vi "main.vi"() -> ()   [LabVIEW 2019]
uses:
  startup_FSM.ctl
  dc_ps_FSM.ctl
  datalog.ctl
  current_ramp_FSM.ctl
  <vilib>/Analysis/6fits.llb/Curve Fitting Criteria.ctl
  <vilib>/Analysis/NI_AALPro.lvlib
  <vilib>/gmath/NI_Gmath.lvlib
panel:
  out "X":dbl[](array[numeric])=[250.0, 300.0, 350.0, 400.0, 450.0, 500.0, 550.0, 600.0, 650.0, 700.0]
  out "points":cluster{"Array":dbl[], "Mean":dbl[]}
  out "Mean":dbl[](array[numeric])
  out "NewVal 5":bool
  in  "appended path":path
  in  "?":T1(tab)
  out "Numeric":dbl min=0.0 max=1.0 step=0.005
  out "Digital Flow Measurements":waveform(dbl)(graph)
  in  "ADJUST":bool
  out "DATA LOG LED":bool
  out "DATA LOG":string
  in  "VOLTAGE":bool
  in  "RESET & CLEAR":bool
  in  "READ ERROR":bool
  in  "Next":bool
  in  "CURRENT LIMIT [A]":dbl(slide)=0.5 min=0.0 max=1.0 step=0.05 scale=0.0..1.0
  in  "OUTPUT CHANNEL":enum32{"Channel 1", "Channel 2", "Channel 3"}(radio)
  in  "STEP":dbl=0.10000000000000002 min=0.05 max=0.5 step=0.05
  out "Slide":dbl(slide) scale=0.0..100.0
  in  "CURRENT RAMP":bool
  in  "POWER SUPPLY STATUS":bool
  in  "Read Button":bool
  in  "Knob":dbl(knob) min=0.0 max=1.0 step=0.005 scale=0.0..1.0
  in  "GPIB ADDRESS":string(combo)="2"
  in  "SERIAL PORT":string(combo)="COM5"
  in  "Command Box":string(combo)
  out "SAMPLE  COUNT":dbl
  out "flow meas":dbl caption="FLOW RATE [SLPM]"
  in  "SAMP. FREQ. [HZ]":dbl=1.0 min=1.0 max=2.5 step=0.5
  in  "New Script":bool
  in  "Clear Buffer":bool
  in  "Connect Button":bool
  in  "Save As Button":bool
  in  "BAUD":string(combo)="9600" caption="BAUD RATE (BIT/S)"
  in  "Start DAQ 2":bool
  in  "Start DAQ":bool
  in  "Stop DAQ":bool
  in  "Configuration":T2={"Sampling"={"Samples per channel"=0, "Sample rate"=0.0}, "Acquisition"={"physical channels"="", "sample mode"=enum."Hardware Timed Single Point", "Min Val."=0.0, "Max Val."=0.0}}
  out "Analogue Flow Measurements":waveform(dbl)(graph)
  out "Coefficients":dbl[](array[numeric])=[-3.1117144499904428, 0.02542890920743523, -2.6853289603939732e-05, 1.2947146249008665e-08]
  in  "Show Curve":bool=TRUE
  in  "Show Points":bool=TRUE
  in  "Load Data":bool
  out "appended array":cluster{"X Values":dbl[], "Y Values":dbl[]}[](graph)=[{"X Values"=[250.0, 300.0, 350.0, 400.0, 450.0, 500.0, 550.0, 600.0, 650.0, 700.0], "Y Values"=[1.805424999999999, 2.3810990099009968, 3.0371608910891195, 3.656717821782189, 4.100871287128724, 4.4772945544554315, 4.869299504950476, 5.299580000000001, 5.624591584158401, 5.9728574999999875]}, {"X Values"=[250.00018963565154, 295.000164139512, 340.0000282955542, 385.00004256878935, 430.00026277216773, 475.00029313870596, 520.0001594137282, 565.0001288827434, 610.0004242971758, 655.0001368461951, 700.0004476537845], "Y Values"=[1.7622871059542533, 2.3768000375757894, 2.9289624170767077, 3.425856115012801, 3.874559922213396, 4.282148677197654, 4.6557018474018514, 5.0023004682122965, 5.3290247161472895, 5.642946889493036, 5.951154061007404]}]
  out "Formula":string="y =  -3.1117 + 0.0254*x - 2.6853E-5*x^2 + 1.2947E-8*x^3"
  out "MSE":dbl=0.0014069661559321211
  in  "Poly Order":i32=3 min=2 max=4 step=1
  in  "Array":bool[](array[boolean])=[FALSE, FALSE, TRUE, FALSE]
  in  "FIT Button":bool caption="Fit"
  in  "base path":path=path "C:/Users/anton/myUnisannio/magistrale/MAPI/esame/acquisizioni"
  # "OUTPUT CURRENT [A]"
  # "POWER SUPPLY \nCONTROLS"
  # "0V"
  # "12V"
  # "A"
  # "linear"
  # "exp"
  # "poly"
  # "power"
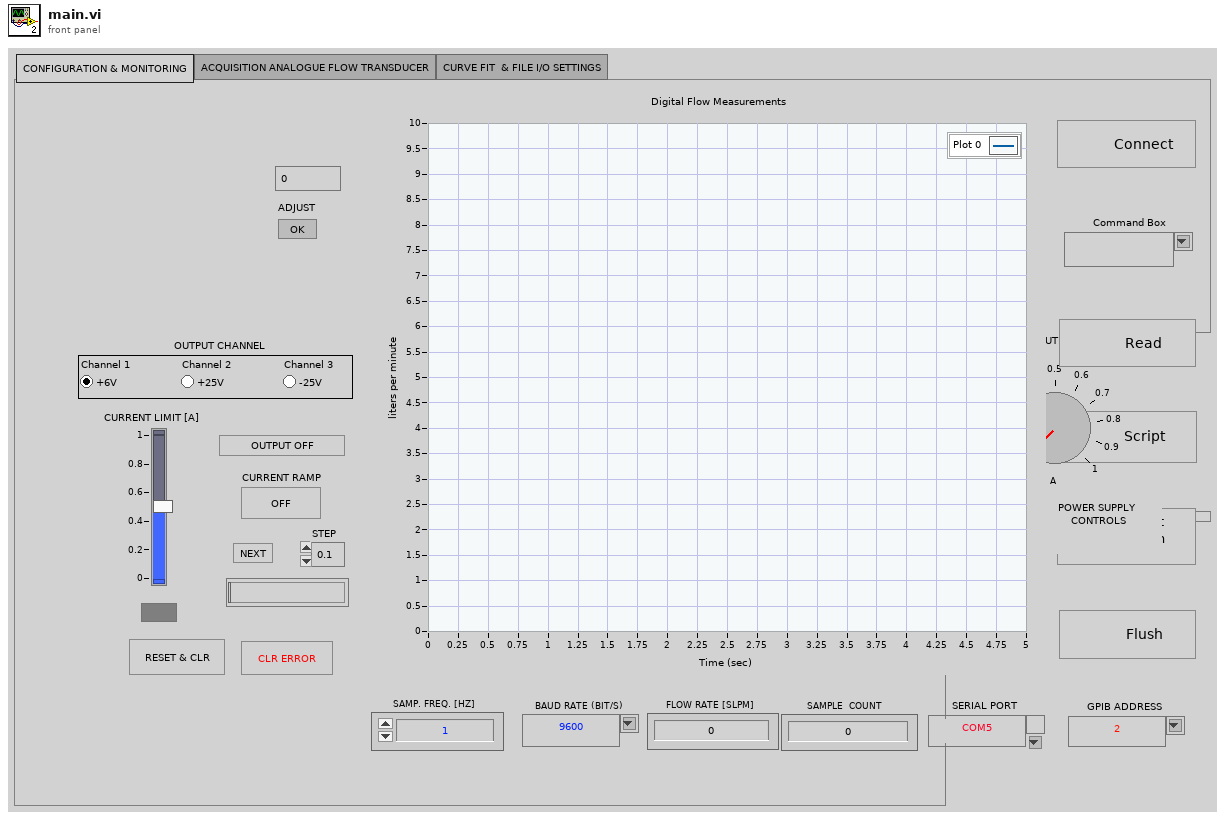
[diagram p1: front panel]
types:
  T1 = enum32{"CONFIGURATION & MONITORING", "ACQUISITION ANALOGUE FLOW TRANSDUCER", "CURVE FIT  & FILE I/O SETTINGS"}
  T2 = cluster{"Sampling":cluster{"Samples per channel":i32, "Sample rate":dbl}, "Acquisition":cluster{"physical channels":tag, "sample mode":enum16{"Finite Samples", "Continuous Samples", "Hardware Timed Single Point"}, "Min Val.":dbl, "Max Val.":dbl}}
  T3 = enum16{"", "Initialize", "Wait", "Shutdown", "Configure", "Read"}
  T4 = enum8{"Enabled", "Disabled", "Disabled and Grayed Out"}
  T5 = typedef "current_ramp_FSM.ctl" = enum16{"STATUS UPDATE", "INIT", "ERROR", "RAMP SETUP", "RAMP ENABLE", "RAMP DISABLE", "RAMP UP", "RAMP DOWN"}
  T6 = typedef "datalog.ctl" = enum16{"Error", "Read Script", "Play Script", "Changed Baud", "Changed Samp. Freq.", "Read All", "Changed Meas Unit", "Print Waveform", "Ramp Disabled", "Ramp Enabled", "Changed Ramp Step", "Changed Output Channel", "Read Error Power Supply", "Reset Power Supply", "DC Output OFF", "DC Output ON", "Connected Arduino", "Disconnected Arduino", "Disable", "Enable", "Changed Port", "Clear DL", "Changed DC Volt", "Changed Out Curr", "Stop Timer", "Start Timer", "Changed Max. Curr."}
  T7 = typedef "dc_ps_FSM.ctl" = enum16{"RESET", "VOLTAGE 12", "VOLTAGE 0", "INIT", "IDLE", "OUTPUT OFF", "OUTPUT ON", "OUT CURR", "SELECT CH", "LIMITS", "ENABLE RAMP", "RAMP UP", "RAMP DOWN", "RAMP STEP", "MEAS", "MEAS?", "ERROR", "READ ERROR", "DISABLE RAMP"}
  T8 = typedef "startup_FSM.ctl" = enum16{"IDLE", "INIT", "START MEAS", "READ", "STOP MEAS", "CHANGE BAUD", "CHANGE SAMP. FREQ.", "CHANGE PORT", "WRITE", "DISCONNECT", "CONNECT", "OUTPUT OFF", "MEAS_UNIT_L", "MEAS_UNIT_mL", "ERROR", "CLEAR BUFF", "OUTPUT ON"}
  T9 = enum16{"Linear", "Polynomial", "Exponential", "Power"}
  T10 = typedef "NI_AALPro.lvlib/Curve Fitting Criteria.ctl" = u16
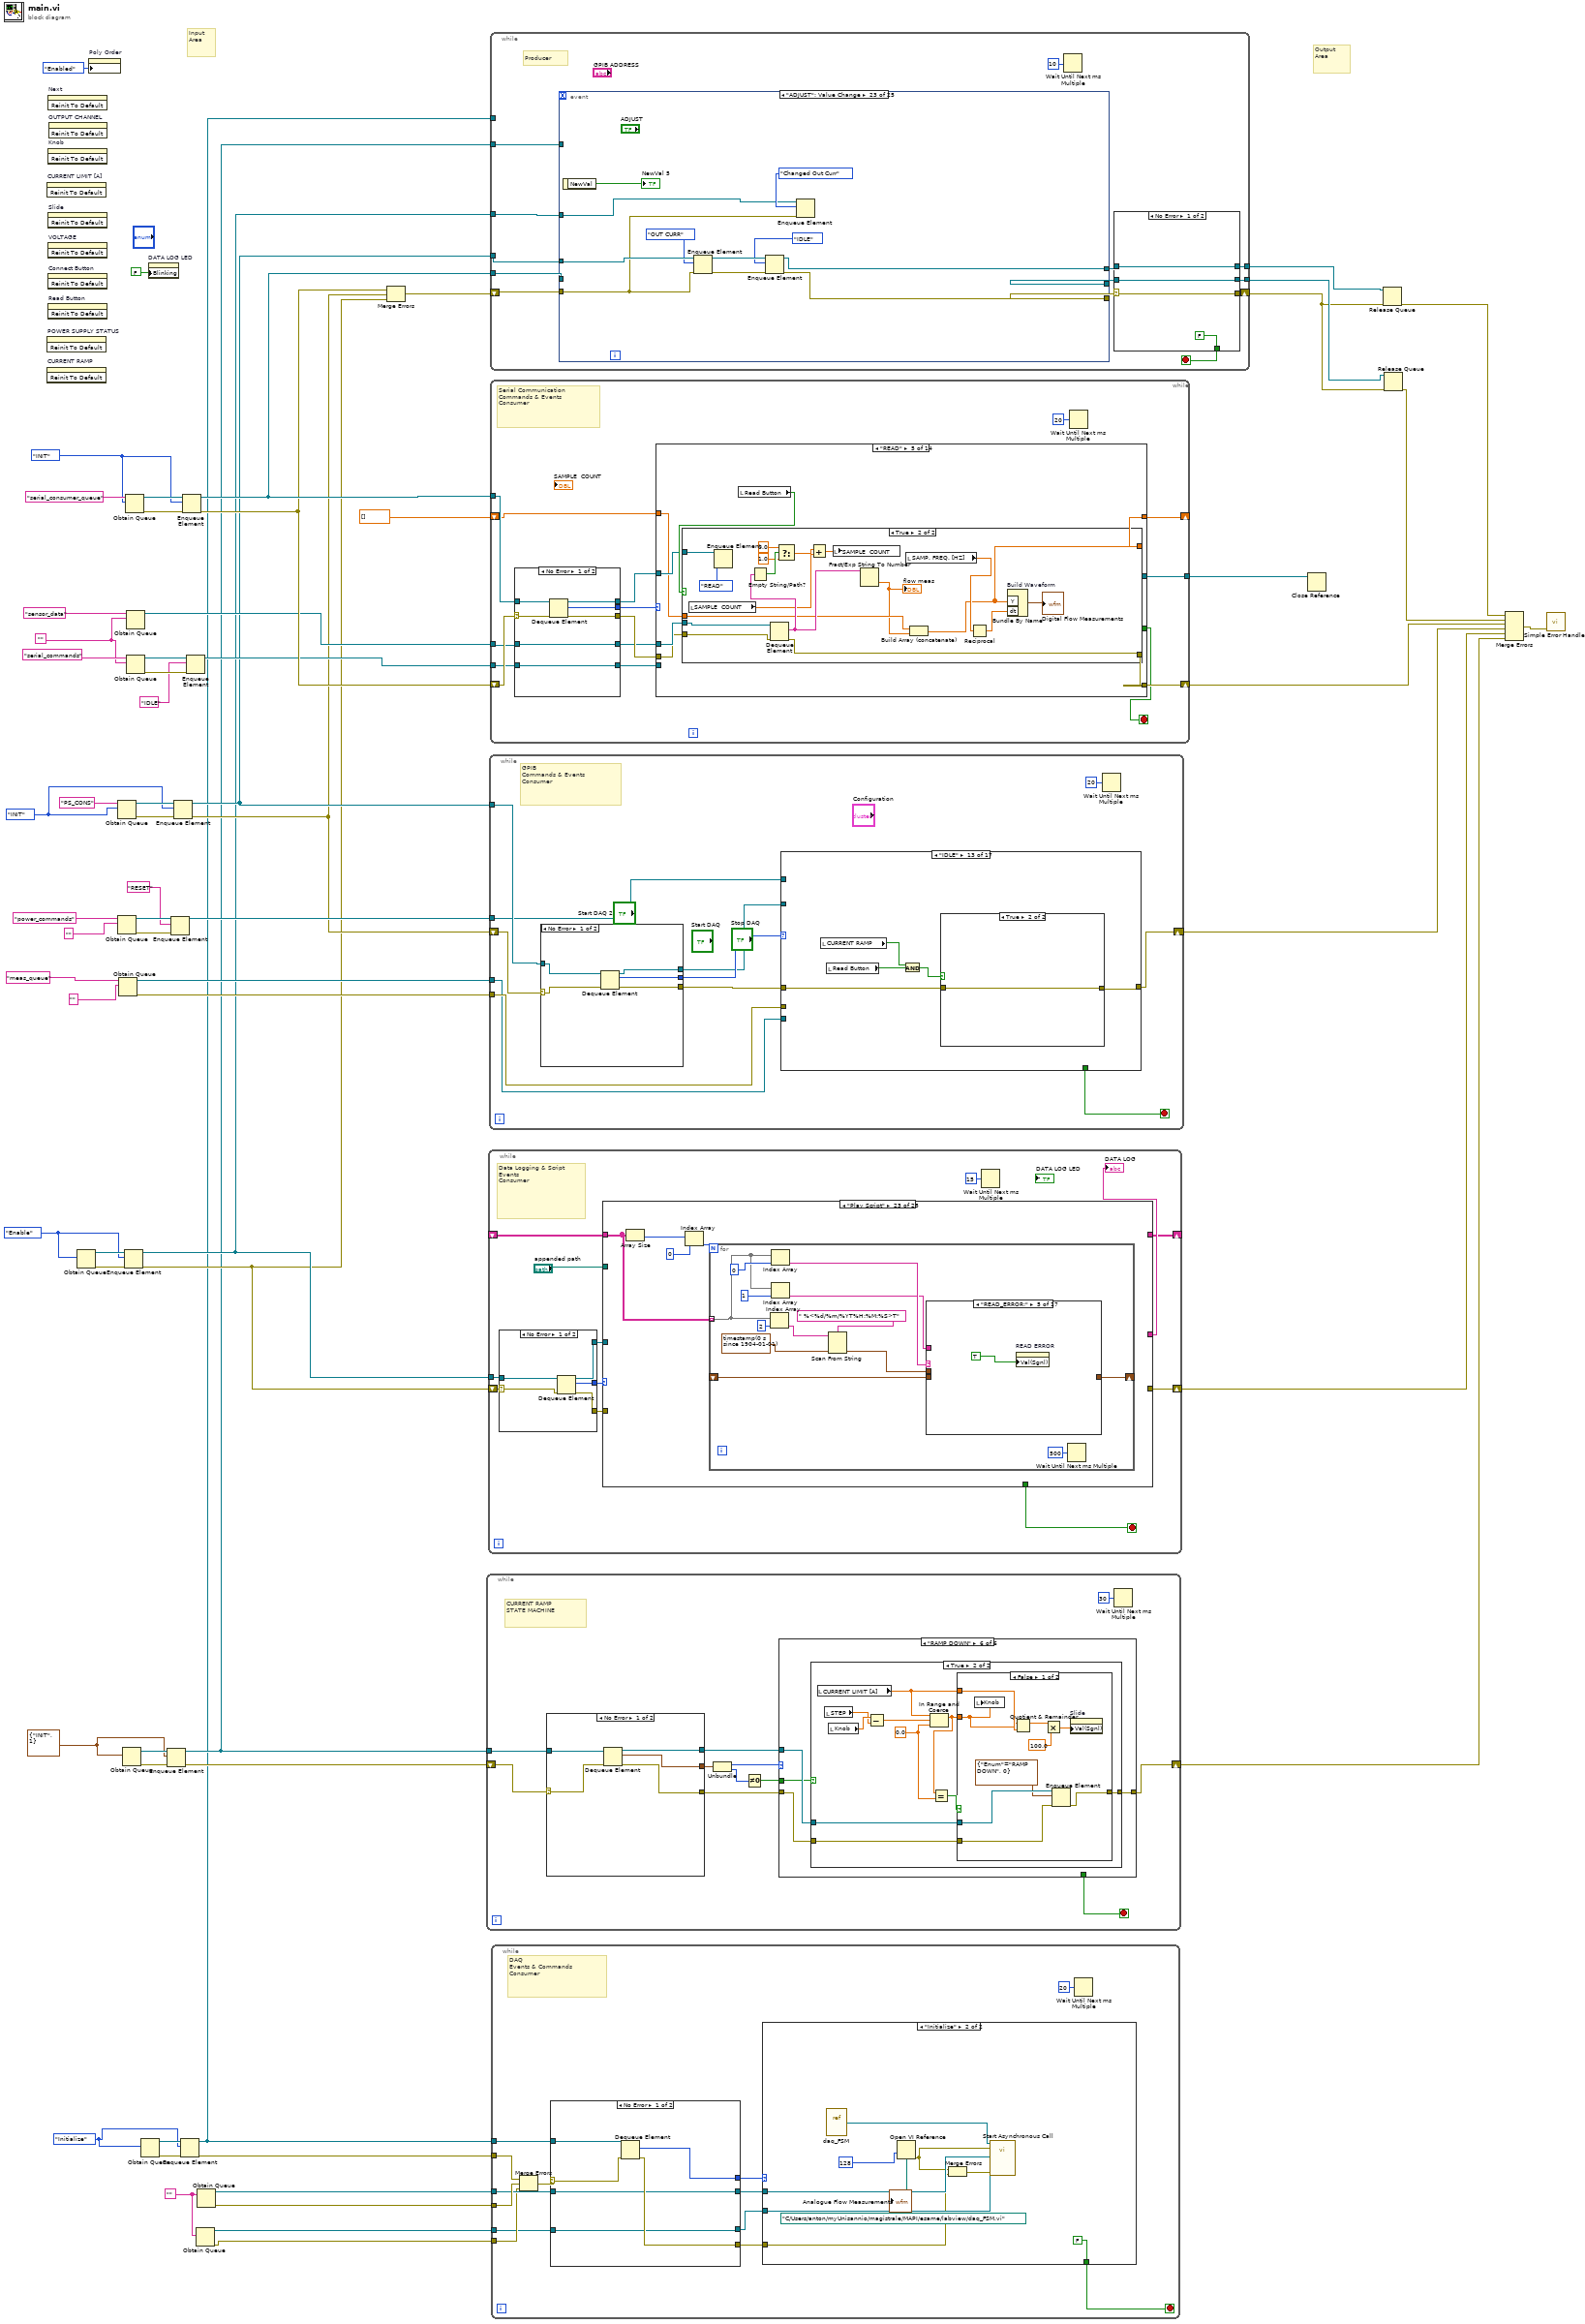
[diagram p0: block diagram]
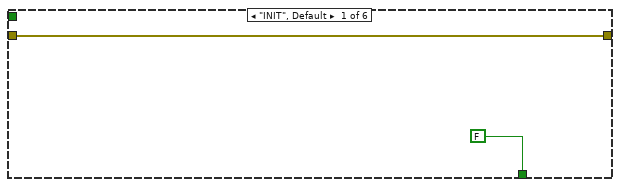
[diagram p4: hidden frame]
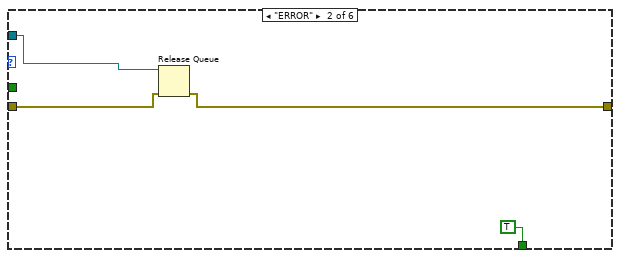
[diagram p5: hidden frame]
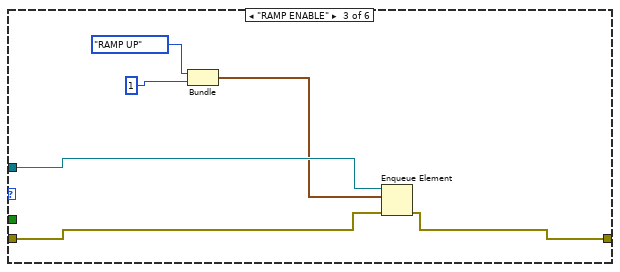
[diagram p6: hidden frame]
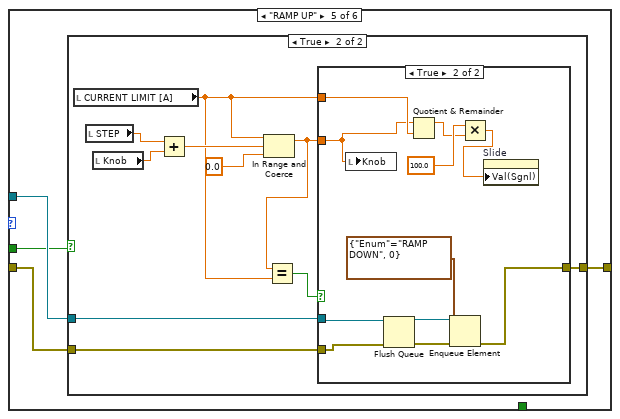
[diagram p8: hidden frame]
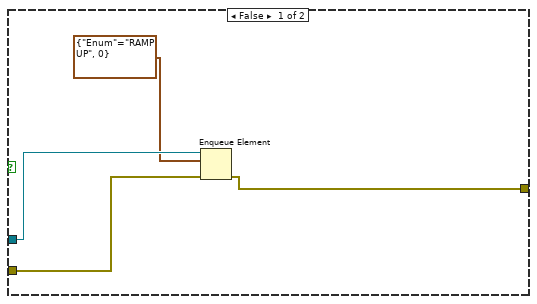
[diagram p9: hidden frame]
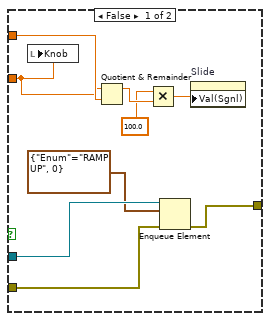
[diagram p10: hidden frame]
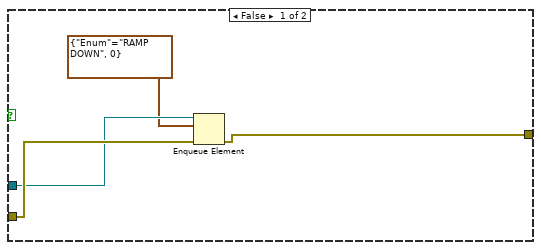
[diagram p11: hidden frame]
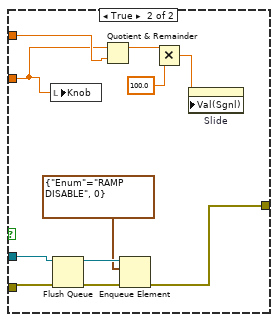
[diagram p12: hidden frame]
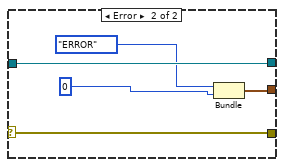
[diagram p13: hidden frame]
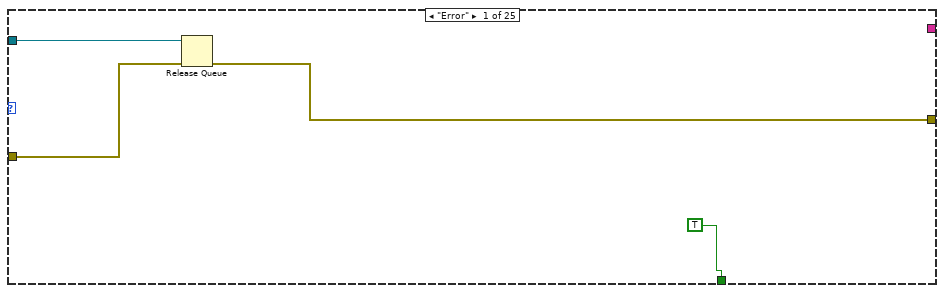
[diagram p14: hidden frame]
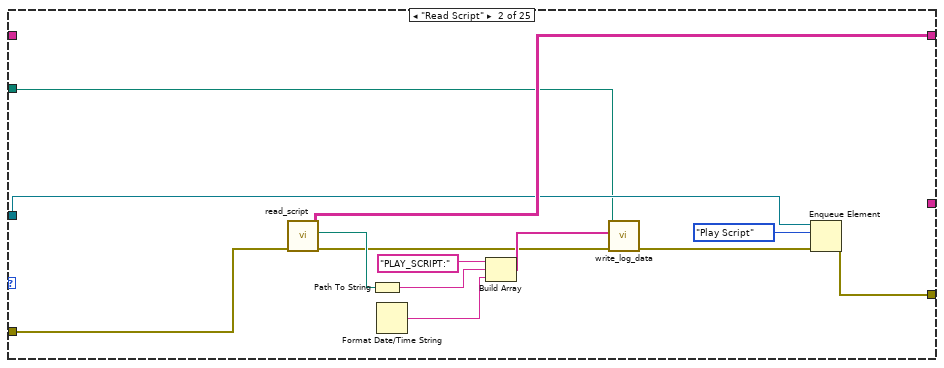
[diagram p15: hidden frame]
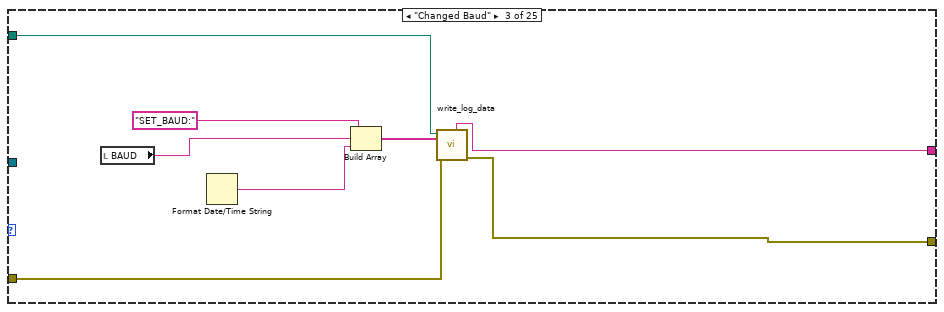
[diagram p16: hidden frame]
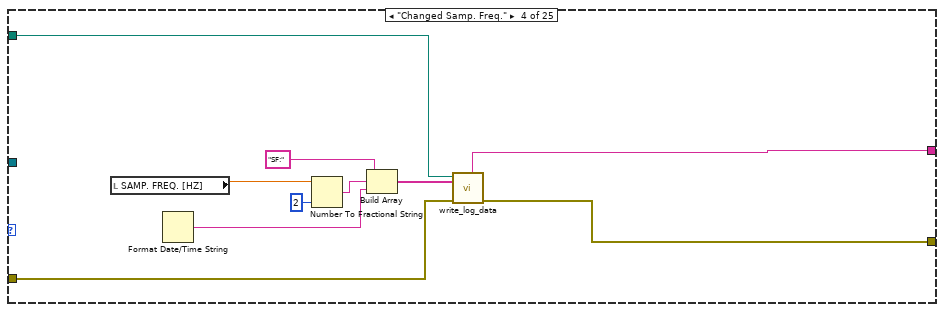
[diagram p17: hidden frame]
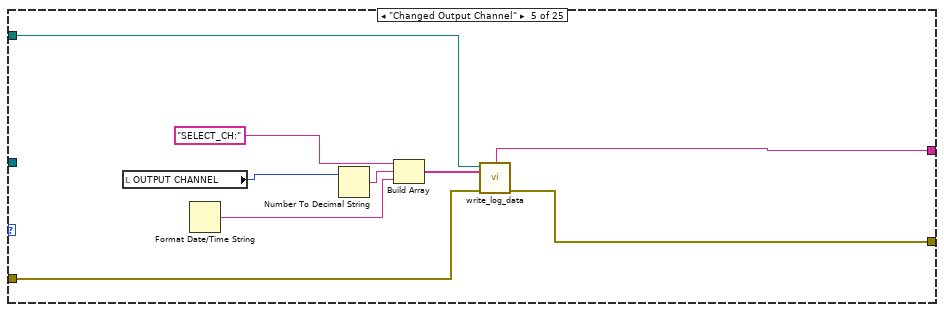
[diagram p18: hidden frame]
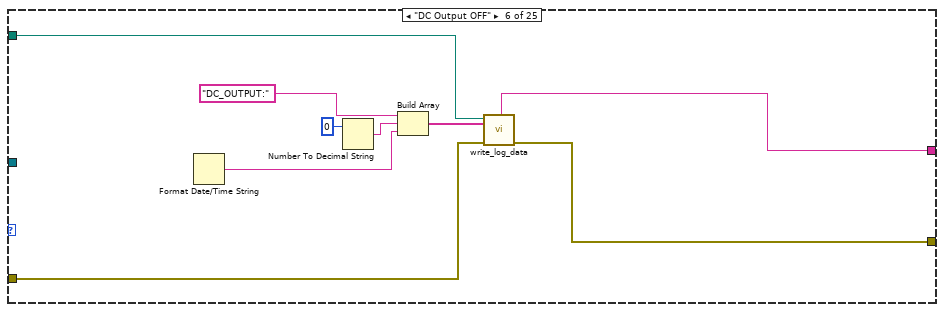
[diagram p19: hidden frame]
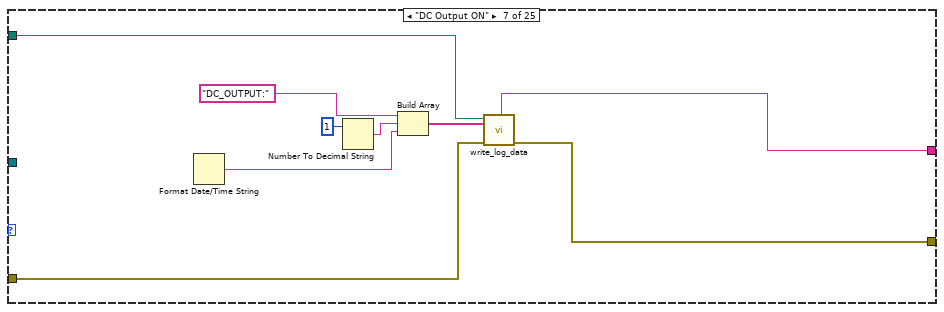
[diagram p20: hidden frame]
diagram:
  w1 = ""
  w8 = T3."Initialize" ("Enum")
  w16 = cluster{"Enum":T5, i32} {"Enum"=enum."INIT", 1} ("error constant")
  w25 = datalog."Enable" ("Enum")
  w44 = dc_ps_FSM."INIT" ("DC Power Supply FSM")
  w15 = ""
  w56 = startup_FSM."INIT" ("element")
  # "Output\nArea"
  # "Input\nArea"
  n1 = invoke on="CURRENT LIMIT [A]" class="Slide (strict)" method="Reinit To Default"() -> ()  [unwired: 3 in, 3 out]
  n2 = invoke on="POWER SUPPLY STATUS" class="Bool (strict)" method="Reinit To Default"() -> ()  [unwired: 3 in, 3 out]
  n3 = invoke on="CURRENT RAMP" class="Bool (strict)" method="Reinit To Default"() -> ()  [unwired: 3 in, 3 out]
  n4 = invoke on="Next" class="Bool (strict)" method="Reinit To Default"() -> ()  [unwired: 3 in, 3 out]
  n5 = invoke on="Knob" class="Knob (strict)" method="Reinit To Default"() -> ()  [unwired: 3 in, 3 out]
  n6 = invoke on="Slide" class="Slide (strict)" method="Reinit To Default"() -> ()  [unwired: 3 in, 3 out]
  n7 = invoke on="VOLTAGE" class="Bool (strict)" method="Reinit To Default"() -> ()  [unwired: 3 in, 3 out]
  n8 = invoke on="Connect Button" class="Bool (strict)" method="Reinit To Default"() -> ()  [unwired: 3 in, 3 out]
  n9 = invoke on="Read Button" class="Bool (strict)" method="Reinit To Default"() -> ()  [unwired: 3 in, 3 out]
  n10 = invoke on="OUTPUT CHANNEL" class="RadioBtnsControl (strict)" method="Reinit To Default"() -> ()  [unwired: 3 in, 3 out]
  n11 = Obtain Queue(element data type=w25) -> (queue out=w26:refnum<queue>, error out=w24:errorcluster)  [unwired: 4 in, 1 out]
  n12 = property on="Poly Order" class="DigNum (strict)"("DisabledEnum"=T4."Enabled" ("Disabled")) -> ()  [unwired: 2 in, 2 out]
  n13 = Obtain Queue(name (unnamed)="PS_CONS", element data type=w44) -> (queue out=w60:refnum<queue>, error out=w59:errorcluster)  [unwired: 3 in, 1 out]
  n14 = Obtain Queue(name (unnamed)="power_commands", element data type="") -> (queue out=w46:refnum<queue>, error out=w47:errorcluster)  [unwired: 3 in, 1 out]
  n15 = Obtain Queue(name (unnamed)="meas_queue", element data type="") -> (queue out=w39:refnum<queue>, error out=w38:errorcluster)  [unwired: 3 in, 1 out]
  n16 = Obtain Queue(element data type=w16) -> (queue out=w20:refnum<queue>, error out=w19:errorcluster)  [unwired: 4 in, 1 out]
  n17 = Enqueue Element(queue=w26, element=w25, error in (no error)=w24) -> (queue out=w23:refnum<queue>, error out=w22:errorcluster)  [unwired: 1 in, 1 out]
  n18 = Obtain Queue(name (unnamed)="serial_consumer_queue", element data type=w56) -> (queue out=w64:refnum<queue>, error out=w63:errorcluster)  [unwired: 3 in, 1 out]
  n19 = Obtain Queue(name (unnamed)="sensor_data", element data type=w15) -> (queue out=w40:refnum<queue>)  [unwired: 3 in, 2 out]
  n20 = Obtain Queue(name (unnamed)="serial_commands", element data type=w15) -> (queue out=w51:refnum<queue>, error out=w53:errorcluster)  [unwired: 3 in, 1 out]
  n21 = Obtain Queue(element data type=w8) -> (queue out=w10:refnum<queue>, error out=w9:errorcluster)  [unwired: 4 in, 1 out]
  n22 = property on="DATA LOG LED" class="Bool (strict)"("Blinking"=FALSE) -> ()  [unwired: 2 in, 2 out]
  n23 = Enqueue Element(queue=w20, element=w16, error in (no error)=w19) -> (queue out=w17:refnum<queue>, error out=w18:errorcluster)  [unwired: 1 in, 1 out]
  n24 = Enqueue Element(queue=w46, element="RESET", error in (no error)=w47) -> (queue out=w43:refnum<queue>)  [unwired: 1 in, 2 out]
  n25 = Enqueue Element(queue=w60, element=w44, error in (no error)=w59) -> (queue out=w37:refnum<queue>, error out=w28:errorcluster)  [unwired: 1 in, 1 out]
  n26 = Enqueue Element(queue=w10, element=w8, error in (no error)=w9) -> (queue out=w5:refnum<queue>, error out=w7:errorcluster)  [unwired: 1 in, 1 out]
  n27 = Enqueue Element(queue=w64, element=w56, error in (no error)=w63) -> (queue out=w62:refnum<queue>, error out=w58:errorcluster)  [unwired: 1 in, 1 out]
  n28 = Enqueue Element(queue=w51, element="IDLE", error in (no error)=w53) -> (queue out=w50:refnum<queue>)  [unwired: 1 in, 2 out]
  n29 = Obtain Queue(element data type=w1) -> (queue out=w3:refnum<queue>, error out=w2:errorcluster)  [unwired: 4 in, 1 out]
  n30 = Obtain Queue(element data type=w1) -> (queue out=w4:refnum<queue>, error out=w6:errorcluster)  [unwired: 4 in, 1 out]
  n31 = Merge Errors(w58, w28, w22) -> (w57:errorcluster)
  n32 = while {
    shift-right: [w72] -> w12
    shift-left: w18 -> [w74]
    tunnel: w17 -> [w75]
    stop <- w70 stop-if-true
    # "CURRENT RAMP \nSTATE MACHINE"
    n33 = case shown="No Error" w74 {
      selector: w74 -> [w169 w174]
      tunnel: w75 -> [w170 w175]
      tunnel: [w168 w174] -> w73
      tunnel: [w167 w175] -> w71
      tunnel: [w166 w173] -> w69
      frame No Error {
        n34 = Dequeue Element(queue=w170, error in (no error)=w169) -> (queue out=w167:refnum<queue>, element=w166:cluster{"Enum":T5, i32}, error out=w168:errorcluster)  [unwired: 1 in, 1 out]
      }
      frame Error {
        n35 = Bundle("Enum"=current_ramp_FSM."ERROR", 0) -> (w173:cluster{"Enum":T5, i32})  [unwired: 1 in]
      }
    }
    n36 = Unbundle(w69) -> ("Enum"=w68:T5, w66:i32)
    n37 = Not Equal To 0?(x=w66) -> (x != 0?=w67:bool)
    n38 = case shown="\"RAMP DOWN\"" w68 {
      tunnel: w73 -> [w78 w81 w87 w89 w92 w130]
      tunnel: [w78 w80 w86 w89 w91 w129] -> w72
      tunnel: w71 -> [_ w82 w88 _ w93 w131]
      tunnel: [FALSE TRUE _ _ _ _] -> w70
      tunnel: w67 -> [_ _ _ _ w90 w128]
      frame "INIT", Default {
      }
      frame "ERROR" {
        n39 = Release Queue(queue=w82, error in (no error)=w81) -> (error out=w80:errorcluster)  [unwired: 1 in, 2 out]
      }
      frame "RAMP ENABLE" {
        n40 = Bundle("element"=current_ramp_FSM."RAMP UP", 1) -> (w83:cluster{"element":T5, i32})  [unwired: 1 in]
        n41 = Enqueue Element(queue=w88, element=w83, error in (no error)=w87) -> (error out=w86:errorcluster)  [unwired: 1 in, 2 out]
      }
      frame "RAMP DISABLE" {
      }
      frame "RAMP UP" {
        n42 = case shown="True" w90 {
          tunnel: w93 -> [w97 w107]
          tunnel: w92 -> [w96 w106]
          tunnel: [w94 w98] -> w91
          frame False {
            n43 = Enqueue Element(queue=w97, element=cluster{"Enum":T5, i32} {"Enum"=enum."RAMP UP", 0}, error in (no error)=w96) -> (error out=w94:errorcluster)  [unwired: 1 in, 2 out]
          }
          frame True {
            n44 = local read "CURRENT LIMIT [A]"() -> (w99:dbl)
            n45 = local read "STEP"() -> (w105:dbl)
            n46 = local read "Knob"() -> (w104:dbl)
            n47 = Add(x=w105, y=w104) -> (x+y=w103:dbl)
            n48 = In Range and Coerce(upper limit=w99, x=w103, lower limit=0.0) -> (coerced(x)=w100:dbl)  [unwired: 1 out]
            n49 = Equal?(x=w100, y=w99) -> (x = y?=w101:bool)
            n50 = case shown="True" w101 {
              tunnel: w107 -> [w109 w122]
              tunnel: w106 -> [w110 w121]
              tunnel: w100 -> [w114 w123]
              tunnel: w99 -> [w115 w127]
              tunnel: [w111 w117] -> w98
              frame False {
                n51 = local write "Knob"(w114) -> ()
                n52 = Quotient & Remainder(x=w114, y=w115) -> (x-y*floor(x/y)=w113:dbl)  [unwired: 1 out]
                n53 = Multiply(x=100.0 ("y"), y=w113) -> (x*y=w116:dbl)
                n54 = Enqueue Element(queue=w109, element=cluster{"Enum":T5, i32} {"Enum"=enum."RAMP UP", 0}, error in (no error)=w110) -> (error out=w111:errorcluster)  [unwired: 1 in, 2 out]
                n55 = property on="Slide" class="Slide (strict)"("Val(Sgnl)"=w116) -> ()  [unwired: 2 in, 2 out]
              }
              frame True {
                n56 = local write "Knob"(w123) -> ()
                n57 = Flush Queue(queue=w122, error in (no error)=w121) -> (queue out=w120:refnum<queue>, error out=w119:errorcluster)  [unwired: 1 out]
                n58 = Quotient & Remainder(x=w123, y=w127) -> (x-y*floor(x/y)=w125:dbl)  [unwired: 1 out]
                n59 = Enqueue Element(queue=w120, element=cluster{"Enum":T5, i32} {"Enum"=enum."RAMP DOWN", 0}, error in (no error)=w119) -> (error out=w117:errorcluster)  [unwired: 1 in, 2 out]
                n60 = Multiply(x=100.0 ("y"), y=w125) -> (x*y=w124:dbl)
                n61 = property on="Slide" class="Slide (strict)"("Val(Sgnl)"=w124) -> ()  [unwired: 2 in, 2 out]
              }
            }
          }
        }
      }
      frame "RAMP DOWN" {
        n62 = case shown="True" w128 {
          tunnel: w131 -> [w134 w145]
          tunnel: w130 -> [w135 w144]
          tunnel: [w132 w139] -> w129
          frame False {
            n63 = Enqueue Element(queue=w134, element=cluster{"Enum":T5, i32} {"Enum"=enum."RAMP DOWN", 0}, error in (no error)=w135) -> (error out=w132:errorcluster)  [unwired: 1 in, 2 out]
          }
          frame True {
            w138 = 0.0 ("lower limit")
            n64 = local read "CURRENT LIMIT [A]"() -> (w140:dbl)
            n65 = local read "STEP"() -> (w136:dbl)
            n66 = local read "Knob"() -> (w137:dbl)
            n67 = Subtract(x=w137, y=w136) -> (x-y=w143:dbl)
            n68 = In Range and Coerce(upper limit=w140, x=w143, lower limit=w138) -> (coerced(x)=w141:dbl)  [unwired: 1 out]
            n69 = Equal?(x=w141, y=w138) -> (x = y?=w142:bool)
            n70 = case shown="False" w142 {
              tunnel: w145 -> [w147 w160]
              tunnel: w144 -> [w148 w159]
              tunnel: w141 -> [w152 w161]
              tunnel: w140 -> [w153 w162]
              tunnel: [w149 w155] -> w139
              frame False {
                n71 = local write "Knob"(w152) -> ()
                n72 = Quotient & Remainder(x=w152, y=w153) -> (x-y*floor(x/y)=w151:dbl)  [unwired: 1 out]
                n73 = Multiply(x=w151, y=100.0) -> (x*y=w154:dbl)
                n74 = Enqueue Element(queue=w147, element=cluster{"Enum":T5, i32} {"Enum"=enum."RAMP DOWN", 0}, error in (no error)=w148) -> (error out=w149:errorcluster)  [unwired: 1 in, 2 out]
                n75 = property on="Slide" class="Slide (strict)"("Val(Sgnl)"=w154) -> ()  [unwired: 2 in, 2 out]
              }
              frame True {
                n76 = local write "Knob"(w161) -> ()
                n77 = Flush Queue(queue=w160, error in (no error)=w159) -> (queue out=w158:refnum<queue>, error out=w157:errorcluster)  [unwired: 1 out]
                n78 = Quotient & Remainder(x=w161, y=w162) -> (x-y*floor(x/y)=w165:dbl)  [unwired: 1 out]
                n79 = Enqueue Element(queue=w158, element=cluster{"Enum":T5, i32} {"Enum"=enum."RAMP DISABLE", 0}, error in (no error)=w157) -> (error out=w155:errorcluster)  [unwired: 1 in, 2 out]
                n80 = Multiply(x=w165, y=100.0) -> (x*y=w163:dbl)
                n81 = property on="Slide" class="Slide (strict)"("Val(Sgnl)"=w163) -> ()  [unwired: 2 in, 2 out]
              }
            }
          }
        }
      }
    }
    n82 = Wait Until Next ms Multiple(millisecond multiple=u32 30) -> ()  [unwired: 1 out]
  }
  n83 = while {
    tunnel: w23 -> [w186]
    shift-right: [w182] -> w13
    shift-left: w22 -> [w187]
    shift-right: [w177] -> _
    shift-left: _ -> [w176]
    stop <- w181 stop-if-true
    # "Data Logging & Script\nEvents\nConsumer"
    n84 = case shown="No Error" w187 {
      selector: w187 -> [w475 w477]
      tunnel: w186 -> [w476 w478]
      tunnel: [w474 datalog."Error" ("Enum")] -> w185
      tunnel: [w473 w478] -> w184
      tunnel: [w472 w477] -> w183
      frame No Error {
        n85 = Dequeue Element(queue=w476, error in (no error)=w475) -> (queue out=w473:refnum<queue>, element=w474:T6, error out=w472:errorcluster)  [unwired: 1 in, 1 out]
      }
      frame Error {
      }
    }
    n86 = case shown="\"Play Script\"" w185 {
      tunnel: w184 -> [w191 w203 _ _ _ _ _ _ _ _ _ w288 w300 _ _ _ _ _ _ _ _ _ _ _ _]
      tunnel: w183 -> [w190 w202 w207 w218 w225 w234 w243 w250 w263 w270 w279 w287 w299 w315 w325 w337 w343 w353 w363 w373 w384 w392 _ w463 w470]
      tunnel: [w189 w192 w205 w216 w223 w233 w242 w251 w261 w269 w278 w286 w298 w313 w323 w335 w345 w352 w362 w371 w382 w390 _ _ _] -> w182
      tunnel: "appended path" -> [_ w200 w212 w219 w226 w235 w244 w253 w264 w271 w280 _ _ w320 w329 w341 w350 w354 w370 w374 w385 w393 _ w464 w471]
      tunnel: [TRUE _ _ _ _ _ _ _ _ _ _ FALSE FALSE _ _ _ _ _ _ _ _ _ _ _ _] -> w181
      tunnel: [_ _ w206 w217 w224 w232 w241 w252 w262 w268 w277 _ _ w314 w324 w336 w344 w351 w361 w372 w383 w391 _ w458 w465] -> w179
      tunnel: [_ w204 _ _ _ _ _ _ _ _ _ _ _ _ _ _ _ _ _ _ _ _ _ _ _] -> w177
      tunnel: w176 -> [_ _ _ _ _ _ _ _ _ _ _ _ _ _ _ _ _ _ _ _ _ _ w397 _ _]
      frame "Error" {
        n87 = Release Queue(queue=w191, error in (no error)=w190) -> (error out=w189:errorcluster)  [unwired: 1 in, 2 out]
      }
      frame "Read Script" {
        n88 = call "read_script.vi"("error in (no error)"=w202) -> ("error out"=w194:errorcluster, "file path"=w198:path, "all rows"=w204:string[][])  [unwired: 8 in]
        n89 = Path To String(path=w198) -> (string=w197:string)
        n90 = Format Date/Time String() -> (date/time string=w196:string)  [unwired: 3 in]
        n91 = Build Array("PLAY_SCRIPT:", w197, w196) -> (w195:string[])
        n92 = call "write_log_data.vi"("error in (no error)"=w194, "Array in"=w195, "appended path"=w200) -> ("error out"=w193:errorcluster)  [unwired: 4 in, 4 out]
        n93 = Enqueue Element(queue=w203, element=datalog."Play Script", error in (no error)=w193) -> (error out=w192:errorcluster)  [unwired: 1 in, 2 out]
      }
      frame "Changed Baud" {
        n94 = local read "BAUD"() -> (w210:string)
        n95 = Format Date/Time String() -> (date/time string=w209:string)  [unwired: 3 in]
        n96 = Build Array("SET_BAUD:", w210, w209) -> (w208:string[])
        n97 = call "write_log_data.vi"("error in (no error)"=w207, "Array in"=w208, "appended path"=w212) -> ("error out"=w205:errorcluster, "data"=w206:string)  [unwired: 4 in, 3 out]
      }
      frame "Changed Samp. Freq." {
        n98 = local read "SAMP. FREQ. [HZ]"() -> (w221:dbl)
        n99 = Format Date/Time String() -> (date/time string=w213:string)  [unwired: 3 in]
        n100 = Number To Fractional String(number=w221, precision (6)=i16 2) -> (F-format string=w222:string)  [unwired: 2 in]
        n101 = Build Array("SF:" ("element"), w222, w213) -> (w220:string[])
        n102 = call "write_log_data.vi"("error in (no error)"=w218, "Array in"=w220, "appended path"=w219) -> ("error out"=w216:errorcluster, "data"=w217:string)  [unwired: 4 in, 3 out]
      }
      frame "Changed Output Channel" {
        n103 = local read "OUTPUT CHANNEL"() -> (w231:enum32{"Channel 1", "Channel 2", "Channel 3"})
        n104 = Format Date/Time String() -> (date/time string=w229:string)  [unwired: 3 in]
        n105 = Number To Decimal String(number=w231) -> (decimal integer string=w230:string)  [unwired: 1 in]
        n106 = Build Array("SELECT_CH:" ("element"), w230, w229) -> (w227:string[])
        n107 = call "write_log_data.vi"("error in (no error)"=w225, "Array in"=w227, "appended path"=w226) -> ("error out"=w223:errorcluster, "data"=w224:string)  [unwired: 4 in, 3 out]
      }
      frame "DC Output OFF" {
        n108 = Format Date/Time String() -> (date/time string=w237:string)  [unwired: 3 in]
        n109 = Number To Decimal String(number=0) -> (decimal integer string=w239:string)  [unwired: 1 in]
        n110 = Build Array("DC_OUTPUT:" ("element"), w239, w237) -> (w236:string[])
        n111 = call "write_log_data.vi"("error in (no error)"=w234, "Array in"=w236, "appended path"=w235) -> ("error out"=w233:errorcluster, "data"=w232:string)  [unwired: 4 in, 3 out]
      }
      frame "DC Output ON" {
        n112 = Format Date/Time String() -> (date/time string=w246:string)  [unwired: 3 in]
        n113 = Number To Decimal String(number=1) -> (decimal integer string=w248:string)  [unwired: 1 in]
        n114 = Build Array("DC_OUTPUT:" ("element"), w248, w246) -> (w245:string[])
        n115 = call "write_log_data.vi"("error in (no error)"=w243, "Array in"=w245, "appended path"=w244) -> ("error out"=w242:errorcluster, "data"=w241:string)  [unwired: 4 in, 3 out]
      }
      frame "Clear DL" {
        n116 = Format Date/Time String() -> (date/time string=w257:string)  [unwired: 3 in]
        n117 = Build Array("CLEAR_BUFF:" ("element"), "1" ("element"), w257) -> (w254:string[])
        n118 = call "write_log_data.vi"("error in (no error)"=w250, "Array in"=w254, "appended path"=w253) -> ("error out"=w251:errorcluster, "data"=w252:string)  [unwired: 4 in, 3 out]
      }
      frame "Read All" {
        n119 = local read "Read Button"() -> (w260:bool)
        n120 = Boolean To (0,1)(Boolean=w260) -> (0, 1=w259:i16)
        n121 = Number To Decimal String(number=w259) -> (decimal integer string=w258:string)  [unwired: 1 in]
        n122 = Format Date/Time String() -> (date/time string=w267:string)  [unwired: 3 in]
        n123 = Build Array("READ_ALL:" ("element"), w258, w267) -> (w265:string[])
        n124 = call "write_log_data.vi"("error in (no error)"=w263, "Array in"=w265, "appended path"=w264) -> ("error out"=w261:errorcluster, "data"=w262:string)  [unwired: 4 in, 3 out]
      }
      frame "Connected Arduino" {
        n125 = Format Date/Time String() -> (date/time string=w273:string)  [unwired: 3 in]
        n126 = Number To Decimal String(number=1) -> (decimal integer string=w275:string)  [unwired: 1 in]
        n127 = Build Array("SERIAL:" ("element"), w275, w273) -> (w272:string[])
        n128 = call "write_log_data.vi"("error in (no error)"=w270, "Array in"=w272, "appended path"=w271) -> ("error out"=w269:errorcluster, "data"=w268:string)  [unwired: 4 in, 3 out]
      }
      frame "Disconnected Arduino" {
        n129 = Format Date/Time String() -> (date/time string=w282:string)  [unwired: 3 in]
        n130 = Number To Decimal String(number=0) -> (decimal integer string=w284:string)  [unwired: 1 in]
        n131 = Build Array("SERIAL:" ("element"), w284, w282) -> (w281:string[])
        n132 = call "write_log_data.vi"("error in (no error)"=w279, "Array in"=w281, "appended path"=w280) -> ("error out"=w278:errorcluster, "data"=w277:string)  [unwired: 4 in, 3 out]
      }
      frame "Disable" {
        n133 = Release Queue(queue=w288, error in (no error)=w287) -> (error out=w286:errorcluster)  [unwired: 1 in, 2 out]
      }
      frame "Enable", Default {
        # "why using default datalog structure/functions when you can create your own!"
        n134 = Get Date/Time In Seconds() -> (seconds since 1Jan1904=w305:timestamp)
        n135 = Format Date/Time String(time format string (%c)="%m%d%Y_%H%M%S", seconds (now)=w305) -> (date/time string=w303:string)  [unwired: 1 in]
        n136 = Concatenate Strings("dl_" ("string"), w303, ".csv" ("string")) -> (w291:string)
        n137 = call "File Dialog"("start path"=path "C:/Users/anton/myUnisannio/magistrale/MAPI/esame/datalogs" ("base path"), "prompt"="Would you like to create a datalog?", "button label"="YES", "default name"=w291) -> ("selected path"=w296:path, "cancelled"=w293:bool, "error out"=w292:errorcluster)  [unwired: 8 in, 1 out]
        n138 = call <vilib>:"Clear Errors.vi"("error in (no error)"=w292) -> ()  [unwired: 5 in, 2 out]
        n139 = case shown="True" w293 {
          tunnel: w300 -> [_ w312]
          tunnel: w299 -> [w307 w311]
          tunnel: [w307 w310] -> w298
          tunnel: w296 -> [w308 _]
          frame False {
            n140 = local write "appended path"(w308) -> ()
            n141 = property on="DATA LOG LED" class="Bool (strict)"("Blinking"=TRUE) -> ()  [unwired: 2 in, 2 out]
          }
          frame True {
            n142 = Enqueue Element(queue=w312, element=datalog."Disable", error in (no error)=w311) -> (error out=w310:errorcluster)  [unwired: 1 in, 2 out]
          }
        }
      }
      frame "Changed Port" {
        n143 = local read "SERIAL PORT"() -> (w318:string)
        n144 = Format Date/Time String() -> (date/time string=w317:string)  [unwired: 3 in]
        n145 = Build Array("SET_PORT:", w318, w317) -> (w316:string[])
        n146 = call "write_log_data.vi"("error in (no error)"=w315, "Array in"=w316, "appended path"=w320) -> ("error out"=w313:errorcluster, "data"=w314:string)  [unwired: 4 in, 3 out]
      }
      frame "Changed DC Volt" {
        n147 = local read "VOLTAGE"() -> (w322:bool)
        n148 = Format Date/Time String() -> (date/time string=w327:string)  [unwired: 3 in]
        n149 = case shown="True" w322 {
          tunnel: ["0" "12"] -> w321
          frame False {
          }
          frame True {
          }
        }
        n150 = Build Array("SOURCE_VOLT:", w321, w327) -> (w326:string[])
        n151 = call "write_log_data.vi"("error in (no error)"=w325, "Array in"=w326, "appended path"=w329) -> ("error out"=w323:errorcluster, "data"=w324:string)  [unwired: 4 in, 3 out]
      }
      frame "Changed Max. Curr." {
        n152 = local read "CURRENT LIMIT [A]"() -> (w334:dbl)
        n153 = Format Date/Time String() -> (date/time string=w339:string)  [unwired: 3 in]
        n154 = Number To Fractional String(number=w334, precision (6)=i16 4) -> (F-format string=w332:string)  [unwired: 2 in]
        n155 = Build Array("SOURCE_CURR:", w332, w339) -> (w338:string[])
        n156 = call "write_log_data.vi"("error in (no error)"=w337, "Array in"=w338, "appended path"=w341) -> ("error out"=w335:errorcluster, "data"=w336:string)  [unwired: 4 in, 3 out]
      }
      frame "Print Waveform" {
        n157 = invoke on="Digital Flow Measurements" class="WFGraph (strict)" method="Export Data to Excel"(error in=w343) -> (error out=w342:errorcluster)  [unwired: 2 in, 2 out]
        n158 = Format Date/Time String() -> (date/time string=w347:string)  [unwired: 3 in]
        n159 = Build Array("EXPORT_GRAPH:", "1" ("element"), w347) -> (w346:string[])
        n160 = call "write_log_data.vi"("error in (no error)"=w342, "Array in"=w346, "appended path"=w350) -> ("error out"=w345:errorcluster, "data"=w344:string)  [unwired: 4 in, 3 out]
      }
      frame "Ramp Enabled" {
        n161 = local read "CURRENT RAMP"() -> (w359:bool)
        n162 = Boolean To (0,1)(Boolean=w359) -> (0, 1=w358:i16)
        n163 = Number To Decimal String(number=w358) -> (decimal integer string=w357:string)  [unwired: 1 in]
        n164 = Format Date/Time String() -> (date/time string=w356:string)  [unwired: 3 in]
        n165 = Build Array("RAMP_ENABLE:", w357, w356) -> (w355:string[])
        n166 = call "write_log_data.vi"("error in (no error)"=w353, "Array in"=w355, "appended path"=w354) -> ("error out"=w352:errorcluster, "data"=w351:string)  [unwired: 4 in, 3 out]
      }
      frame "Changed Ramp Step" {
        n167 = local read "STEP"() -> (w367:dbl)
        n168 = Format Date/Time String() -> (date/time string=w369:string)  [unwired: 3 in]
        n169 = Number To Fractional String(number=w367, precision (6)=i16 2) -> (F-format string=w366:string)  [unwired: 2 in]
        n170 = Build Array("RAMP_STEP:", w366, w369) -> (w364:string[])
        n171 = call "write_log_data.vi"("error in (no error)"=w363, "Array in"=w364, "appended path"=w370) -> ("error out"=w362:errorcluster, "data"=w361:string)  [unwired: 4 in, 3 out]
      }
      frame "Changed Out Curr" {
        n172 = local read "Knob"() -> (w378:dbl)
        n173 = Number To Fractional String(number=w378, precision (6)=i16 4) -> (F-format string=w377:string)  [unwired: 2 in]
        n174 = Format Date/Time String() -> (date/time string=w376:string)  [unwired: 3 in]
        n175 = Build Array("OUT_CURR:", w377, w376) -> (w375:string[])
        n176 = call "write_log_data.vi"("error in (no error)"=w373, "Array in"=w375, "appended path"=w374) -> ("error out"=w371:errorcluster, "data"=w372:string)  [unwired: 4 in, 3 out]
      }
      frame "Read Error Power Supply" {
        n177 = Format Date/Time String() -> (date/time string=w387:string)  [unwired: 3 in]
        n178 = Build Array("READ_ERROR:", "1" ("element"), w387) -> (w386:string[])
        n179 = call "write_log_data.vi"("error in (no error)"=w384, "Array in"=w386, "appended path"=w385) -> ("error out"=w382:errorcluster, "data"=w383:string)  [unwired: 4 in, 3 out]
      }
      frame "Reset Power Supply" {
        n180 = Format Date/Time String() -> (date/time string=w395:string)  [unwired: 3 in]
        n181 = Build Array("RESET_PS:", "1" ("element"), w395) -> (w394:string[])
        n182 = call "write_log_data.vi"("error in (no error)"=w392, "Array in"=w394, "appended path"=w393) -> ("error out"=w390:errorcluster, "data"=w391:string)  [unwired: 4 in, 3 out]
      }
      frame "Play Script" {
        n183 = Array Size(array=w397) -> (size(s)=w399:i32[])
        n184 = Index Array "Index Array"(array=w399, index=0) -> (element=w398:i32)
        n185 = for {
          N: w398 -> [_]
          tunnel: w397 -> [w409] mode=indexing
          shift-right: [w402] -> _
          shift-left: _ -> [w403]
          n186 = Index Array(array=w409, index=2) -> (element=w406:string)
          n187 = Index Array(array=w409, index=0) -> (element=w411:string)
          n188 = Index Array(array=w409, index=1) -> (element=w410:string)
          n189 = Scan From String(format string=" %<%d/%m/%YT%H:%M:%S>T", input string=w406, default 1=timestamp(0 s since 1904-01-01)) -> (output 1=w404:timestamp)  [unwired: 2 in, 3 out]
          n190 = case shown="\"READ_ERROR:\"" w411 {
            tunnel: w410 -> [w414 w416 w419 w421 _ w426 w428 w431 _ w435 w439 _ w441 w444 w447 _ w457]
            tunnel: w404 -> [_ _ _ _ _ _ _ _ _ _ _ _ _ _ w449 _ _]
            tunnel: w403 -> [_ _ _ _ _ _ _ _ _ _ _ _ _ _ w448 _ _]
            tunnel: [_ _ _ _ _ _ _ _ _ _ _ _ _ _ w445 _ _] -> w402
            frame "SF:" {
              n191 = Fract/Exp String To Number(string=w414) -> (number=w415:dbl)  [unwired: 3 in, 1 out]
              n192 = property on="SAMP. FREQ. [HZ]" class="DigNum (strict)"("Val(Sgnl)"=w415) -> ()  [unwired: 2 in, 2 out]
            }
            frame "SOURCE_VOLT:" {
              n193 = Decimal String To Number(string=w416) -> (number=w418:i32)  [unwired: 2 in, 1 out]
              n194 = Not Equal To 0?(x=w418) -> (x != 0?=w417:bool)
              n195 = property on="VOLTAGE" class="Bool (strict)"("Val(Sgnl)"=w417) -> ()  [unwired: 2 in, 2 out]
            }
            frame "SOURCE_CURR:" {
              n196 = Fract/Exp String To Number(string=w419) -> (number=w420:dbl)  [unwired: 3 in, 1 out]
              n197 = property on="CURRENT LIMIT [A]" class="Slide (strict)"("Val(Sgnl)"=w420) -> ()  [unwired: 2 in, 2 out]
            }
            frame "OUT_CURR:" {
              n198 = Fract/Exp String To Number(string=w421) -> (number=w422:dbl)  [unwired: 3 in, 1 out]
              n199 = flat-sequence {
                tunnel: w422 -> [w423]
                frame #0 {
                  n200 = property on="Knob" class="Knob (strict)"("Val(Sgnl)"=w423) -> ()  [unwired: 2 in, 2 out]
                }
                frame #1 {
                  n201 = property on="ADJUST" class="Bool (strict)"("Val(Sgnl)"=TRUE) -> ()  [unwired: 2 in, 2 out]
                }
              }
            }
            frame "READ_ERROR:" {
              n202 = property on="READ ERROR" class="Bool (strict)"("Val(Sgnl)"=TRUE) -> ()  [unwired: 2 in, 2 out]
            }
            frame "SELECT_CH:" {
              n203 = Decimal String To Number(string=w426) -> (offset past number=w427:i32)  [unwired: 2 in, 1 out]
              n204 = property on="OUTPUT CHANNEL" class="RadioBtnsControl (strict)"("Val(Sgnl)"=w427) -> ()  [unwired: 2 in, 2 out]
            }
            frame "DC_OUTPUT:" {
              n205 = Decimal String To Number(string=w428) -> (number=w430:i32)  [unwired: 2 in, 1 out]
              n206 = Not Equal To 0?(x=w430) -> (x != 0?=w429:bool)
              n207 = property on="POWER SUPPLY STATUS" class="Bool (strict)"("Val(Sgnl)"=w429) -> ()  [unwired: 2 in, 2 out]
            }
            frame "SERIAL:" {
              n208 = Decimal String To Number(string=w431) -> (number=w432:i32)  [unwired: 2 in, 1 out]
              n209 = Not Equal To 0?(x=w432) -> (x != 0?=w433:bool)
              n210 = property on="Connect Button" class="Bool (strict)"("Val(Sgnl)"=w433) -> ()  [unwired: 2 in, 2 out]
            }
            frame "RESET_PS:" {
              n211 = property on="RESET & CLEAR" class="Bool"("Val(Sgnl)"=TRUE) -> ()  [unwired: 2 in, 2 out]
            }
            frame "RAMP_STEP:" {
              n212 = Fract/Exp String To Number(string=w435) -> (number=w436:dbl)  [unwired: 3 in, 1 out]
              n213 = property on="STEP" class="DigNum (strict)"("Val(Sgnl)"=w436) -> ()  [unwired: 2 in, 2 out]
            }
            frame "RAMP_ENABLE:" {
              n214 = Decimal String To Number(string=w439) -> (number=w438:i32)  [unwired: 2 in, 1 out]
              n215 = Not Equal To 0?(x=w438) -> (x != 0?=w437:bool)
              n216 = property on="CURRENT RAMP" class="Bool (strict)"("Val(Sgnl)"=w437) -> ()  [unwired: 2 in, 2 out]
            }
            frame "EXPORT_GRAPH" {
              n217 = property on="Save As Button" class="Bool (strict)"("Val(Sgnl)"=TRUE ("Value (Signaling)")) -> ()  [unwired: 2 in, 2 out]
            }
            frame "SET_BAUD:", Default {
              n218 = property on="BAUD" class="CmbBox"("Val(Sgnl)"=w441) -> ()  [unwired: 2 in, 2 out]
            }
            frame "READ_ALL:" {
              n219 = Decimal String To Number(string=w444) -> (number=w442:i32)  [unwired: 2 in, 1 out]
              n220 = Not Equal To 0?(x=w442) -> (x != 0?=w443:bool)
              n221 = property on="Read Button" class="Bool (strict)"("Val(Sgnl)"=w443) -> ()  [unwired: 2 in, 2 out]
            }
            frame "TIMER:" {
              n222 = Decimal String To Number(string=w447) -> (number=w446:i32)  [unwired: 2 in, 1 out]
              n223 = case shown="1" w446 {
                tunnel: w449 -> [w454 w455]
                tunnel: w448 -> [w453 _]
                tunnel: [_ w455] -> w445
                frame 0, Default {
                  n224 = Subtract(x=w454, y=w453) -> (x-y=w452:dbl)
                  n225 = Multiply(x=w452, y=1000.0) -> (x*y=w450:dbl)
                  n226 = Wait Until Next ms Multiple(millisecond multiple=w450) -> ()  [unwired: 1 out]
                }
                frame 1 {
                }
              }
            }
            frame "CLEAR_BUFF:" {
              n227 = property on="Clear Buffer" class="Bool (strict)"("Val(Sgnl)"=TRUE ("Value (Signaling)")) -> ()  [unwired: 2 in, 2 out]
            }
            frame "SET_PORT:" {
              n228 = property on="SERIAL PORT" class="CmbBox"("Val(Sgnl)"=w457) -> ()  [unwired: 2 in, 2 out]
            }
          }
          n229 = Wait Until Next ms Multiple(millisecond multiple=u32 500 ("milliseconds to wait")) -> ()  [unwired: 1 out]
        }
      }
      frame "Start Timer" {
        n230 = Format Date/Time String() -> (date/time string=w462:string)  [unwired: 3 in]
        n231 = Build Array("TIMER:" ("element"), "1" ("element"), w462) -> (w459:string[])
        n232 = call "write_log_data.vi"("error in (no error)"=w463, "Array in"=w459, "appended path"=w464) -> ("data"=w458:string)  [unwired: 4 in, 4 out]
      }
      frame "Stop Timer" {
        n233 = Format Date/Time String() -> (date/time string=w469:string)  [unwired: 3 in]
        n234 = Build Array("TIMER:" ("element"), "0" ("element"), w469) -> (w466:string[])
        n235 = call "write_log_data.vi"("error in (no error)"=w470, "Array in"=w466, "appended path"=w471) -> ("data"=w465:string)  [unwired: 4 in, 4 out]
      }
    }
    "DATA LOG" <- w179
    n236 = Wait Until Next ms Multiple(millisecond multiple=u32 15) -> ()  [unwired: 1 out]
  }
  n237 = while {
    tunnel: w43 -> [w485]
    tunnel: w39 -> [w482]
    tunnel: w38 -> [w483]
    tunnel: w37 -> [w489]
    shift-right: [w484] -> w30
    shift-left: w28 -> [w490]
    stop <- w481 stop-if-true
    # "GPIB \nCommands & Events \nConsumer"
    n238 = case shown="No Error" w490 {
      selector: w490 -> [w599 w601]
      tunnel: w489 -> [w600 w602]
      tunnel: [w598 dc_ps_FSM."ERROR" ("DC Power Supply FSM")] -> w488
      tunnel: [w597 w602] -> w487
      tunnel: [w596 w601] -> w486
      frame No Error {
        n239 = Dequeue Element(queue=w600, error in (no error)=w599) -> (queue out=w597:refnum<queue>, element=w598:T7, error out=w596:errorcluster)  [unwired: 1 in, 1 out]
      }
      frame Error {
      }
    }
    n240 = case shown="\"IDLE\"" w488 {
      tunnel: w487 -> [_ _ _ _ _ _ _ _ _ _ _ _ _ _ _ _ _]
      tunnel: w486 -> [w492 w497 w505 w508 w529 w532 w539 _ w548 w554 w567 w571 w574 w582 w585 w590 w593]
      tunnel: w485 -> [w494 w498 w506 w509 w530 w533 w540 _ w549 w551 w568 w572 _ w583 w587 w591 w594]
      tunnel: [w491 w495 w500 w507 w523 _ w534 w541 w546 w553 w562 w569 w573 w580 w584 w589 w592] -> w484
      tunnel: w483 -> [_ _ _ _ _ _ _ w545 _ _ w566 _ _ _ _ _ _]
      tunnel: w482 -> [_ _ _ _ _ _ _ w544 _ w552 w565 _ _ _ _ _ _]
      tunnel: [_ _ _ _ _ _ _ _ _ FALSE TRUE _ _ _ _ _ _] -> w481
      frame "OUTPUT OFF" {
        n241 = Enqueue Element(queue=w494, element="OUTPUT OFF", error in (no error)=w492) -> (error out=w491:errorcluster)  [unwired: 1 in, 2 out]
      }
      frame "OUTPUT ON" {
        n242 = Enqueue Element(queue=w498, element="OUTPUT ON", error in (no error)=w497) -> (error out=w495:errorcluster)  [unwired: 1 in, 2 out]
      }
      frame "OUT CURR" {
        n243 = local read "Knob"() -> (w499:dbl)
        n244 = Number To Fractional String(number=w499, precision (6)=i16 4) -> (F-format string=w504:string)  [unwired: 2 in]
        n245 = Concatenate Strings("CURR " ("element"), w504) -> (w501:string)
        n246 = Enqueue Element(queue=w506, element=w501, error in (no error)=w505) -> (error out=w500:errorcluster)  [unwired: 1 in, 2 out]
      }
      frame "SELECT CH" {
        n247 = case shown="\"Channel 2\", Default" "OUTPUT CHANNEL" {
          tunnel: w509 -> [w514 w518 w522]
          tunnel: w508 -> [w513 w517 w521]
          tunnel: [w511 w515 w519] -> w507
          frame "Channel 1" {
            n248 = Enqueue Element(queue=w514, element="INST P6V", error in (no error)=w513) -> (error out=w511:errorcluster)  [unwired: 1 in, 2 out]
          }
          frame "Channel 2", Default {
            n249 = Enqueue Element(queue=w518, element="INST P25V", error in (no error)=w517) -> (error out=w515:errorcluster)  [unwired: 1 in, 2 out]
          }
          frame "Channel 3" {
            n250 = Enqueue Element(queue=w522, element="INST N25V", error in (no error)=w521) -> (error out=w519:errorcluster)  [unwired: 1 in, 2 out]
          }
        }
      }
      frame "LIMITS" {
        n251 = Number To Fractional String(number="CURRENT LIMIT [A]", precision (6)=i16 4) -> (F-format string=w525:string)  [unwired: 2 in]
        n252 = Concatenate Strings("SOURCE:CURR " ("element"), w525) -> (w528:string)
        n253 = Enqueue Element(queue=w530, element=w528, error in (no error)=w529) -> (error out=w523:errorcluster)  [unwired: 1 in, 2 out]
      }
      frame "ENABLE RAMP" {
        n254 = Enqueue Element(queue=w533, element="RAMP ENABLE", error in (no error)=w532) -> ()  [unwired: 1 in, 3 out]
      }
      frame "RAMP STEP" {
        n255 = Number To Fractional String(number="STEP") -> (F-format string=w536:string)  [unwired: 3 in]
        n256 = Concatenate Strings("RAMP:STEP " ("element"), w536) -> (w538:string)
        n257 = Enqueue Element(queue=w540, element=w538, error in (no error)=w539) -> (error out=w534:errorcluster)  [unwired: 1 in, 2 out]
      }
      frame "MEAS?" {
        n258 = Dequeue Element(queue=w544, error in (no error)=w545) -> (element=w543:string, error out=w541:errorcluster)  [unwired: 1 in, 2 out]
        n259 = Fract/Exp String To Number(string=w543) -> (number=w542:dbl)  [unwired: 3 in, 1 out]
        n260 = local write "SAMPLE  COUNT"(w542) -> ()
      }
      frame "DISABLE RAMP" {
        n261 = Enqueue Element(queue=w549, element="RAMP DISABLE", error in (no error)=w548) -> (error out=w546:errorcluster)  [unwired: 1 in, 2 out]
      }
      frame "INIT", Default {
        n262 = local read "GPIB ADDRESS"() -> (w550:string)
        n263 = vi-ref "power_supply_FSM.vi"() -> (w559:refnum<vi>)
        n264 = Open VI Reference(type specifier VI Refnum (for type only)=w559, vi path=path "C:/Users/anton/myUnisannio/magistrale/MAPI/esame/labview/power_supply_FSM.vi", options=128, error in (no error)=w554) -> (vi reference=w556:refnum<vi>, error out=w555:errorcluster)  [unwired: 2 in]
        n265 = call-by-ref "Start Asynchronous Call"(reference=w556, error in=w555, "measurements q"=w552, "commands q"=w551, "GPIB"=w550) -> (error out=w553:errorcluster)  [unwired: 17 in, 1 out]
      }
      frame "ERROR" {
        n266 = Release Queue(queue=w568, error in (no error)=w567) -> (error out=w564:errorcluster)  [unwired: 1 in, 2 out]
        n267 = Release Queue(queue=w565, error in (no error)=w566) -> (error out=w563:errorcluster)  [unwired: 1 in, 2 out]
        n268 = Merge Errors(w564, w563) -> (w562:errorcluster)
      }
      frame "MEAS" {
        n269 = Enqueue Element(queue=w572, element="MEAS?", error in (no error)=w571) -> (error out=w569:errorcluster)  [unwired: 1 in, 2 out]
      }
      frame "IDLE" {
        n270 = local read "CURRENT RAMP"() -> (w577:bool)
        n271 = local read "Read Button"() -> (w576:bool)
        n272 = And(x=w577, y=w576) -> (x .and. y?=w575:bool)
        n273 = case shown="True" w575 {
          tunnel: [w578 w579] -> w573
          tunnel: w574 -> [w578 w579]
          frame False {
          }
          frame True {
          }
        }
      }
      frame "READ ERROR" {
        n274 = Enqueue Element(queue=w583, element="READ:ERROR", error in (no error)=w582) -> (error out=w580:errorcluster)  [unwired: 1 in, 2 out]
      }
      frame "RESET" {
        n275 = Enqueue Element(queue=w587, element="RESET", error in (no error)=w585) -> (error out=w584:errorcluster)  [unwired: 1 in, 2 out]
      }
      frame "VOLTAGE 12" {
        n276 = Enqueue Element(queue=w591, element="SOURCE:VOLT 12", error in (no error)=w590) -> (error out=w589:errorcluster)  [unwired: 1 in, 2 out]
      }
      frame "VOLTAGE 0" {
        n277 = Enqueue Element(queue=w594, element="SOURCE:VOLT 0", error in (no error)=w593) -> (error out=w592:errorcluster)  [unwired: 1 in, 2 out]
      }
    }
    n278 = Wait Until Next ms Multiple(millisecond multiple=u32 20) -> ()  [unwired: 1 out]
  }
  n279 = while {
    tunnel: w62 -> [w616]
    shift-right: [w614] -> w34
    shift-left: w57 -> [w615]
    tunnel: w37 -> [w613]
    tunnel: [w612] -> w36
    tunnel: [w611] -> w35
    tunnel: w23 -> [w605]
    tunnel: w17 -> [w604]
    tunnel: w5 -> [_]
    stop <- w610 stop-if-true
    # "Producer"
    n280 = event shown="[22] \"ADJUST\": Value Change" {
      selector: _ -> [_ _ _ _ _ _ _ _ _ _ _ _ _ _ _ _ _ _ _ _ _ _ _ _ _]
      dyn-events: _ -> [_ _ _ _ _ _ _ _ _ _ _ _ _ _ _ _ _ _ _ _ _ _ _ _ _]
      timeout: _ -> [_ _ _ _ _ _ _ _ _ _ _ _ _ _ _ _ _ _ _ _ _ _ _ _ _]
      tunnel: w616 -> [w641 w651 w659 w665 _ _ _ _ _ _ _ _ w821 _ _ _ _ _ w913 _ w926 _ _ _ w970]
      tunnel: w615 -> [w633 w643 w658 w662 _ _ _ w767 _ w789 w799 w809 w819 w848 w862 w883 w894 w897 w910 w915 w918 w928 w930 w941 w966]
      tunnel: [w636 w647 w654 w664 _ _ _ w770 _ w793 w803 w812 w817 w847 w864 w886 _ w898 w906 _ w921 w928 w936 w944 w968] -> w609
      tunnel: [w638 w646 w653 w663 _ _ _ _ _ _ _ _ w820 _ _ _ _ _ w905 _ w922 _ _ _ w969] -> w607
      tunnel: w613 -> [_ _ _ _ _ _ _ w775 _ w797 w807 w814 w818 _ w866 w891 _ w903 _ _ _ w929 w939 w948 w972]
      tunnel: [_ _ _ _ _ _ _ w771 _ w795 w805 w813 _ _ w865 _ _ _ _ _ _ w929 w934 w946 w972] -> w608
      tunnel: w605 -> [w634 w644 _ w661 _ _ _ w768 _ w790 w800 w810 w815 _ w861 w885 w893 w896 w911 w916 w919 _ w931 w942 w967]
      tunnel: w604 -> [_ _ _ _ _ _ _ _ _ _ _ _ w816 w849 _ _ _ _ _ _ _ _ _ _ _]
      event "BAUD": Value Change {
        (unwired) "CHANGING THE BIT RATE SET FOR THE SERIAL CONNECTION"
        n281 = event-data() -> ()  [unwired: 1 in, 6 out]
        n282 = Enqueue Element(queue=w634, element=datalog."Changed Baud", error in (no error)=w633) -> ()  [unwired: 1 in, 3 out]
        n283 = Enqueue Element(queue=w641, element=startup_FSM."CHANGE BAUD", error in (no error)=w633) -> (queue out=w639:refnum<queue>, error out=w637:errorcluster)  [unwired: 1 in, 1 out]
        n284 = Enqueue Element(queue=w639, element=startup_FSM."IDLE", error in (no error)=w637) -> (queue out=w638:refnum<queue>, error out=w636:errorcluster)  [unwired: 1 in, 1 out]
      }
      event "SAMP. FREQ. [HZ]": Value Change {
        (unwired) "CHANGING SAMPLING FREQUENCY"
        n285 = event-data() -> ()  [unwired: 1 in, 1 out]
        n286 = Enqueue Element(queue=w644, element=datalog."Changed Samp. Freq.", error in (no error)=w643) -> ()  [unwired: 1 in, 3 out]
        n287 = Enqueue Element(queue=w651, element=startup_FSM."CHANGE SAMP. FREQ.", error in (no error)=w643) -> (queue out=w649:refnum<queue>, error out=w648:errorcluster)  [unwired: 1 in, 1 out]
        n288 = Enqueue Element(queue=w649, element=startup_FSM."IDLE", error in (no error)=w648) -> (queue out=w646:refnum<queue>, error out=w647:errorcluster)  [unwired: 1 in, 1 out]
      }
      event "Command Box": Value Change {
        (unwired) "to be implemented"
        n289 = event-data() -> ()  [unwired: 1 in, 6 out]
        n290 = Enqueue Element(queue=w659, element=startup_FSM."WRITE", error in (no error)=w658) -> (queue out=w656:refnum<queue>, error out=w655:errorcluster)  [unwired: 1 in, 1 out]
        n291 = Enqueue Element(queue=w656, element=startup_FSM."IDLE", error in (no error)=w655) -> (queue out=w653:refnum<queue>, error out=w654:errorcluster)  [unwired: 1 in, 1 out]
      }
      event "Connect Button": Value Change {
        (unwired) "CONNECTING TO ARDUINO"
        n292 = event-data() -> ("NewVal"=w660:bool)  [unwired: 1 in]
        n293 = case shown="False" w660 {
          tunnel: w665 -> [w675 w685]
          tunnel: [w671 w681] -> w664
          tunnel: [w670 w680] -> w663
          tunnel: w662 -> [w668 w678]
          tunnel: w661 -> [w667 w677]
          frame False {
            n294 = Enqueue Element(queue=w667, element=datalog."Disconnected Arduino", error in (no error)=w668) -> ()  [unwired: 1 in, 3 out]
            n295 = Enqueue Element(queue=w675, element=startup_FSM."DISCONNECT", error in (no error)=w668) -> (queue out=w673:refnum<queue>, error out=w672:errorcluster)  [unwired: 1 in, 1 out]
            n296 = Enqueue Element(queue=w673, element=startup_FSM."IDLE", error in (no error)=w672) -> (queue out=w670:refnum<queue>, error out=w671:errorcluster)  [unwired: 1 in, 1 out]
          }
          frame True {
            n297 = Enqueue Element(queue=w677, element=datalog."Connected Arduino", error in (no error)=w678) -> ()  [unwired: 1 in, 3 out]
            n298 = Enqueue Element(queue=w685, element=startup_FSM."CONNECT", error in (no error)=w678) -> (queue out=w683:refnum<queue>, error out=w682:errorcluster)  [unwired: 1 in, 1 out]
            n299 = Enqueue Element(queue=w683, element=startup_FSM."IDLE", error in (no error)=w682) -> (queue out=w680:refnum<queue>, error out=w681:errorcluster)  [unwired: 1 in, 1 out]
          }
        }
      }
      event "Load Data": Value Change {
        n300 = event-data() -> ()  [unwired: 1 in, 6 out]
        n301 = for {
          N: 10 -> [_]
          tunnel: "base path" -> [w706]
          tunnel: [w701] -> w688 mode=indexing
          tunnel: 50.0 ("STEP") -> [w699]
          tunnel: 250 ("x") -> [w698]
          i -> [w700]
          n302 = Multiply(x=w699, y=w700) -> (x*y=w697:dbl)
          n303 = Add(x=w697, y=w698) -> (x+y=w696:dbl)
          n304 = Number To Decimal String(number=w696) -> (decimal integer string=w695:string)  [unwired: 1 in]
          n305 = Concatenate Strings(w695, "_III.csv" ("string")) -> (w692:string)
          n306 = Concatenate Strings(w695, "_I.csv" ("string")) -> (w694:string)
          n307 = Concatenate Strings(w695, "_II.csv" ("string")) -> (w693:string)
          n308 = Concatenate Strings(w695, "_IV.csv" ("string")) -> (w691:string)
          n309 = Build Path(base path=w706, name or relative path=w694) -> (appended path=w710:path)
          n310 = Build Path(base path=w706, name or relative path=w693) -> (appended path=w709:path)
          n311 = Build Path(base path=w706, name or relative path=w692) -> (appended path=w708:path)
          n312 = Build Path(base path=w706, name or relative path=w691) -> (appended path=w707:path)
          n313 = call "curve_fitter.vi"("Path 4"=w707, "Path 3"=w708, "Path 2"=w709, "Path"=w710) -> ("Arithmetic Mean"=w701:dbl)  [unwired: 4 in, 3 out]
        }
        "Mean" <- w688
      }
      event "Show Points": Value Change {
        w712 = dbl[] [250.0, 300.0, 350.0, 400.0, 450.0, 500.0, 550.0, 600.0, 650.0, 700.0] ("Array")
        n314 = event-data() -> ()  [unwired: 1 in, 6 out]
        n315 = local read "Mean"() -> (w713:dbl[])
        n316 = Bundle "Bundle"("Array"=w712, "Mean"=w713) -> (→"points":cluster{"Array":dbl[], "Mean":dbl[]})  [unwired: 1 in]
        "X" <- w712
      }
      event "FIT Button", "Poly Order": Value Change {
        n317 = event-data() -> ()  [unwired: 1 in, 6 out]
        n318 = local read "Array"() -> (w731:bool[])
        n319 = local read "Mean"() -> (w729:dbl[])
        n320 = local read "X"() -> (w724:dbl[])
        n321 = Search 1D Array(1D array=w731, element=TRUE) -> (index of element=w732:i32)  [unwired: 1 in]
        n322 = case shown="0, Default" w732 {
          tunnel: w729 -> [w740 w749 w756 w765]
          tunnel: w724 -> [w739 w748 w755 w764]
          tunnel: [w735 w744 w751 w760] -> w714
          tunnel: [T9."Linear" ("fit type") T9."Power" ("fit type") T9."Polynomial" ("fit type") T9."Exponential" ("fit type")] -> w728
          tunnel: [w733 w742 w752 w758] -> w716
          frame 0, Default {
            w738 = T10 0 items=["Least Square", "Least Absolute Residual", "Bisquare"] ("method")
            n323 = call <vilib>:"Linear Fit.vi"("Y"=w740, "X"=w739, "method"=w738) -> ("slope"=w737:dbl, "intercept"=w736:dbl, "residue"=w733:dbl)  [unwired: 8 in, 2 out]
            n324 = Build Array(w736, w737) -> (w735:dbl[])
          }
          frame 3 {
            w747 = T10 0 items=["Least Square", "Least Absolute Residual", "Bisquare"] ("method")
            n325 = call <vilib>:"Power Fit.vi"("Y"=w749, "X"=w748, "method"=w747) -> ("amplitude"=w746:dbl, "power"=w745:dbl, "offset"=w741:dbl, "residue"=w742:dbl)  [unwired: 7 in, 2 out]
            n326 = Build Array(w745, w746, w741) -> (w744:dbl[])
          }
          frame 2 {
            w754 = T10 0 items=["Least Square", "Least Absolute Residual", "Bisquare"] ("method")
            n327 = local read "Poly Order"() -> (w750:i32)
            n328 = call <vilib>:"General Polynomial Fit.vi"("Y"=w756, "polynomial order"=w750, "X"=w755, "method"=w754) -> ("Polynomial Coefficients"=w751:dbl[], "residue"=w752:dbl)  [unwired: 8 in, 2 out]
          }
          frame 1 {
            w763 = T10 0 items=["Least Square", "Least Absolute Residual", "Bisquare"] ("method")
            n329 = call <vilib>:"Exponential Fit.vi"("Y"=w765, "X"=w764, "method"=w763) -> ("amplitude"=w762:dbl, "damping"=w761:dbl, "offset"=w757:dbl, "residue"=w758:dbl)  [unwired: 7 in, 2 out]
            n330 = Build Array(w761, w762, w757) -> (w760:dbl[])
          }
        }
        "MSE" <- w716
        "Coefficients" <- w714
        n331 = local read "points"() -> (w718:cluster{"Array":dbl[], "Mean":dbl[]})
        n332 = call "Regression Equation String.vi"("coefficients"=w714, "precision"=4, "fit type"=w728) -> ("Formula"=w725:string)  [unwired: 8 in]
        n333 = Array Max & Min(array=w724) -> (max value=w723:dbl, min value=w722:dbl)  [unwired: 2 out]
        n334 = call <vilib>:"Eval y=f(x) Optimal Step.vi"("formula"=w725, "end"=w723, "start"=w722) -> ("Y Values"=w721:dbl[], "X Values"=w720:dbl[])  [unwired: 2 in, 2 out]
        n335 = Concatenate Strings("y = " ("string"), w725) -> (→"Formula":string)
        n336 = Bundle("X Values"=w720, "Y Values"=w721) -> (w719:cluster{"X Values":dbl[], "Y Values":dbl[]})  [unwired: 1 in]
        n337 = Build Array(w718, w719) -> (→"appended array":cluster{"X Values":dbl[], "Y Values":dbl[]}[])
      }
      event "STEP": Value Change {
        n338 = event-data() -> ()  [unwired: 1 in, 6 out]
        n339 = Enqueue Element(queue=w768, element=datalog."Changed Ramp Step", error in (no error)=w767) -> ()  [unwired: 1 in, 3 out]
        n340 = Enqueue Element(queue=w775, element=dc_ps_FSM."RAMP STEP", error in (no error)=w767) -> (queue out=w773:refnum<queue>, error out=w769:errorcluster)  [unwired: 1 in, 1 out]
        n341 = Enqueue Element(queue=w773, element=dc_ps_FSM."IDLE", error in (no error)=w769) -> (queue out=w771:refnum<queue>, error out=w770:errorcluster)  [unwired: 1 in, 1 out]
      }
      event "Array": Value Change {
        n342 = event-data() -> ("OldVal"=w779:bool[])  [unwired: 1 in, 5 out]
        n343 = Search 1D Array(1D array=w779, element=TRUE) -> (index of element=w777:i32)  [unwired: 1 in]
        n344 = case shown="0, Default" w777 {
          selector: w777 -> [w783 _]
          tunnel: "Array" -> [w785 _]
          frame 0, Default {
            n345 = Replace Array Subset(array=w785, new element=FALSE ("new element/subarray"), index=w783) -> (w781:bool[])
            n346 = local write "Array"(w781) -> ()
            n347 = Index Array(array=w781, index=2) -> (element=w780:bool)
            n348 = case shown="False" w780 {
              frame False {
                n349 = property on="Poly Order" class="DigNum (strict)"("DisabledEnum"=T4."Disabled and Grayed Out" ("Disabled")) -> ()  [unwired: 2 in, 2 out]
              }
              frame True {
                n350 = property on="Poly Order" class="DigNum (strict)"("DisabledEnum"=T4."Enabled" ("Disabled")) -> ()  [unwired: 2 in, 2 out]
              }
            }
          }
          frame -1 {
          }
        }
      }
      event "OUTPUT CHANNEL": Value Change {
        n351 = event-data() -> ()  [unwired: 1 in, 6 out]
        n352 = Enqueue Element(queue=w790, element=datalog."Changed Output Channel", error in (no error)=w789) -> ()  [unwired: 1 in, 3 out]
        n353 = Enqueue Element(queue=w797, element=dc_ps_FSM."SELECT CH", error in (no error)=w789) -> (queue out=w796:refnum<queue>, error out=w794:errorcluster)  [unwired: 1 in, 1 out]
        n354 = Enqueue Element(queue=w796, element=dc_ps_FSM."IDLE", error in (no error)=w794) -> (queue out=w795:refnum<queue>, error out=w793:errorcluster)  [unwired: 1 in, 1 out]
      }
      event "READ ERROR": Value Change {
        n355 = event-data() -> ()  [unwired: 1 in, 6 out]
        n356 = Enqueue Element(queue=w807, element=dc_ps_FSM."READ ERROR", error in (no error)=w799) -> (queue out=w806:refnum<queue>, error out=w804:errorcluster)  [unwired: 1 in, 1 out]
        n357 = Enqueue Element(queue=w800, element=datalog."Read Error Power Supply", error in (no error)=w799) -> ()  [unwired: 1 in, 3 out]
        n358 = Enqueue Element(queue=w806, element=dc_ps_FSM."IDLE", error in (no error)=w804) -> (queue out=w805:refnum<queue>, error out=w803:errorcluster)  [unwired: 1 in, 1 out]
      }
      event "RESET & CLEAR": Value Change {
        n359 = event-data() -> ()  [unwired: 1 in, 6 out]
        n360 = Enqueue Element(queue=w810, element=datalog."Reset Power Supply", error in (no error)=w809) -> ()  [unwired: 1 in, 3 out]
        n361 = Enqueue Element(queue=w814, element=dc_ps_FSM."RESET", error in (no error)=w809) -> (queue out=w813:refnum<queue>, error out=w812:errorcluster)  [unwired: 1 in, 1 out]
      }
      event "CURRENT RAMP": Value Change {
        n362 = event-data() -> ("NewVal"=w822:bool)  [unwired: 1 in]
        n363 = case shown="True" w822 {
          tunnel: w821 -> [w829 w841]
          tunnel: w819 -> [w830 w842]
          tunnel: [w829 w841] -> w820
          tunnel: [w830 w837] -> w817
          tunnel: w818 -> [_ w845]
          tunnel: w816 -> [w828 w836]
          tunnel: w815 -> [w827 w835]
          frame False {
            n364 = Enqueue Element(queue=w827, element=datalog."Ramp Enabled") -> ()  [unwired: 2 in, 3 out]
            n365 = Bundle("element"=current_ramp_FSM."RAMP DISABLE", 1) -> (w823:cluster{"element":T5, i32})  [unwired: 1 in]
            n366 = Enqueue Element(queue=w828, element=w823) -> ()  [unwired: 2 in, 3 out]
          }
          frame True {
            n367 = local write "Knob"(0.0 ("Knob")) -> ()
            n368 = Bundle("element"=current_ramp_FSM."RAMP ENABLE", 1) -> (w831:cluster{"element":T5, i32})  [unwired: 1 in]
            n369 = Enqueue Element(queue=w835, element=datalog."Ramp Enabled") -> ()  [unwired: 2 in, 3 out]
            n370 = Enqueue Element(queue=w845, element=dc_ps_FSM."OUT CURR", error in (no error)=w842) -> (queue out=w840:refnum<queue>, error out=w839:errorcluster)  [unwired: 1 in, 1 out]
            n371 = Enqueue Element(queue=w840, element=dc_ps_FSM."IDLE", error in (no error)=w839) -> (error out=w837:errorcluster)  [unwired: 1 in, 2 out]
            n372 = Enqueue Element(queue=w836, element=w831) -> ()  [unwired: 2 in, 3 out]
          }
        }
      }
      event "Next": Value Change {
        n373 = event-data() -> ()  [unwired: 1 in, 1 out]
        n374 = local read "CURRENT RAMP"() -> (w846:bool)
        n375 = case shown="True" w846 {
          tunnel: w849 -> [_ w859]
          tunnel: w848 -> [w850 w858]
          tunnel: [w850 w851] -> w847
          frame False {
          }
          frame True {
            n376 = Preview Queue Element(queue=w859, error in (no error)=w858) -> (queue out=w856:refnum<queue>, element=w857:cluster{"Enum":T5, i32}, error out=w852:errorcluster)  [unwired: 1 in, 1 out]
            n377 = Unbundle(w857) -> ("Enum"=w854:T5)  [unwired: 1 out]
            n378 = Bundle("Enum"=w854, 1) -> (w855:cluster{"Enum":T5, i32})  [unwired: 1 in]
            n379 = Enqueue Element(queue=w856, element=w855, error in (no error)=w852) -> (error out=w851:errorcluster)  [unwired: 1 in, 2 out]
          }
        }
      }
      event "VOLTAGE": Value Change {
        n380 = event-data() -> ("NewVal"=w863:bool)  [unwired: 1 in]
        n381 = case shown="True" w863 {
          tunnel: w866 -> [w873 w881]
          tunnel: [w872 w880] -> w865
          tunnel: w862 -> [w871 w879]
          tunnel: [w869 w877] -> w864
          frame False {
            n382 = Enqueue Element(queue=w873, element=dc_ps_FSM."VOLTAGE 0", error in (no error)=w871) -> (queue out=w874:refnum<queue>, error out=w870:errorcluster)  [unwired: 1 in, 1 out]
            n383 = Enqueue Element(queue=w874, element=dc_ps_FSM."IDLE", error in (no error)=w870) -> (queue out=w872:refnum<queue>, error out=w869:errorcluster)  [unwired: 1 in, 1 out]
          }
          frame True {
            n384 = Enqueue Element(queue=w881, element=dc_ps_FSM."VOLTAGE 12", error in (no error)=w879) -> (queue out=w882:refnum<queue>, error out=w878:errorcluster)  [unwired: 1 in, 1 out]
            n385 = Enqueue Element(queue=w882, element=dc_ps_FSM."IDLE", error in (no error)=w878) -> (queue out=w880:refnum<queue>, error out=w877:errorcluster)  [unwired: 1 in, 1 out]
          }
        }
        n386 = Enqueue Element(queue=w861, element=datalog."Changed DC Volt", error in (no error)=w862) -> ()  [unwired: 1 in, 3 out]
      }
      event "Slide": Value Change {
        n387 = event-data() -> ()  [unwired: 1 in, 1 out]
        n388 = Enqueue Element(queue=w891, element=dc_ps_FSM."OUT CURR", error in (no error)=w883) -> (queue out=w889:refnum<queue>, error out=w888:errorcluster)  [unwired: 1 in, 1 out]
        n389 = Enqueue Element(queue=w889, element=dc_ps_FSM."IDLE", error in (no error)=w888) -> (error out=w886:errorcluster)  [unwired: 1 in, 2 out]
        n390 = Enqueue Element(queue=w885, element=datalog."Changed Out Curr", error in (no error)=w883) -> ()  [unwired: 1 in, 3 out]
      }
      event "Save As Button": Value Change {
        n391 = event-data() -> ()  [unwired: 1 in, 1 out]
        n392 = Enqueue Element(queue=w893, element=datalog."Print Waveform", error in (no error)=w894) -> ()  [unwired: 1 in, 3 out]
      }
      event "CURRENT LIMIT [A]": Value Change {
        n393 = event-data() -> ()  [unwired: 1 in, 2 out]
        n394 = Enqueue Element(queue=w896, element=datalog."Changed Max. Curr.", error in (no error)=w897) -> ()  [unwired: 1 in, 3 out]
        n395 = Enqueue Element(queue=w903, element=dc_ps_FSM."LIMITS", error in (no error)=w897) -> (queue out=w902:refnum<queue>, error out=w899:errorcluster)  [unwired: 1 in, 1 out]
        n396 = Enqueue Element(queue=w902, element=dc_ps_FSM."IDLE", error in (no error)=w899) -> (error out=w898:errorcluster)  [unwired: 1 in, 2 out]
      }
      event "Clear Buffer": Value Change {
        n397 = event-data() -> ()  [unwired: 1 in, 6 out]
        n398 = Enqueue Element(queue=w913, element=startup_FSM."CLEAR BUFF", error in (no error)=w910) -> (queue out=w908:refnum<queue>, error out=w907:errorcluster)  [unwired: 1 in, 1 out]
        n399 = Enqueue Element(queue=w911, element=datalog."Clear DL", error in (no error)=w910) -> ()  [unwired: 1 in, 3 out]
        n400 = Enqueue Element(queue=w908, element=startup_FSM."IDLE", error in (no error)=w907) -> (queue out=w905:refnum<queue>, error out=w906:errorcluster)  [unwired: 1 in, 1 out]
      }
      event "New Script": Value Change {
        n401 = event-data() -> ()  [unwired: 1 in, 1 out]
        n402 = Enqueue Element(queue=w916, element=datalog."Read Script", error in (no error)=w915) -> ()  [unwired: 1 in, 3 out]
      }
      event "SERIAL PORT": Value Change {
        n403 = event-data() -> ()  [unwired: 1 in, 1 out]
        n404 = Enqueue Element At Opposite End(queue=w919, element=datalog."Changed Port", error in (no error)=w918) -> ()  [unwired: 1 in, 3 out]
        n405 = Enqueue Element At Opposite End(queue=w926, element=startup_FSM."CHANGE PORT", error in (no error)=w918) -> (queue out=w924:refnum<queue>, error out=w923:errorcluster)  [unwired: 1 in, 1 out]
        n406 = Enqueue Element At Opposite End(queue=w924, element=startup_FSM."IDLE", error in (no error)=w923) -> (queue out=w922:refnum<queue>, error out=w921:errorcluster)  [unwired: 1 in, 1 out]
      }
      event "Knob": Value Change {
        n407 = event-data() -> ()  [unwired: 1 in, 1 out]
        "Numeric" <- "Knob"
      }
      event "ADJUST": Value Change {
        n408 = event-data() -> ("NewVal"=→"NewVal 5":bool)  [unwired: 1 in]
        n409 = Enqueue Element(queue=w939, element=dc_ps_FSM."OUT CURR", error in (no error)=w930) -> (queue out=w938:refnum<queue>, error out=w937:errorcluster)  [unwired: 1 in, 1 out]
        n410 = Enqueue Element(queue=w938, element=dc_ps_FSM."IDLE", error in (no error)=w937) -> (queue out=w934:refnum<queue>, error out=w936:errorcluster)  [unwired: 1 in, 1 out]
        n411 = Enqueue Element(queue=w931, element=datalog."Changed Out Curr", error in (no error)=w930) -> ()  [unwired: 1 in, 3 out]
      }
      event "POWER SUPPLY STATUS": Value Change {
        n412 = event-data() -> ("NewVal"=w949:bool)  [unwired: 1 in]
        n413 = case shown="False" w949 {
          tunnel: w948 -> [w956 w965]
          tunnel: w941 -> [w953 w964]
          tunnel: [w955 w962] -> w945
          tunnel: [w957 w961] -> w947
          tunnel: w942 -> [w951 w960]
          tunnel: w941 -> [w952 w958]
          frame False {
            n414 = Enqueue Element(queue=w951, element=datalog."DC Output OFF", error in (no error)=w952) -> ()  [unwired: 1 in, 3 out]
            n415 = Enqueue Element(queue=w956, element=dc_ps_FSM."OUTPUT OFF", error in (no error)=w953) -> (queue out=w957:refnum<queue>, error out=w955:errorcluster)  [unwired: 1 in, 1 out]
          }
          frame True {
            n416 = Enqueue Element(queue=w960, element=datalog."DC Output ON", error in (no error)=w958) -> ()  [unwired: 1 in, 3 out]
            n417 = Enqueue Element(queue=w965, element=dc_ps_FSM."OUTPUT ON", error in (no error)=w964) -> (queue out=w961:refnum<queue>, error out=w962:errorcluster)  [unwired: 1 in, 1 out]
          }
        }
        n418 = Enqueue Element(queue=w947, element=dc_ps_FSM."IDLE", error in (no error)=w945) -> (queue out=w946:refnum<queue>, error out=w944:errorcluster)  [unwired: 1 in, 1 out]
      }
      event "Read Button": Value Change {
        n419 = event-data() -> ("NewVal"=w971:bool)  [unwired: 1 in]
        n420 = case shown="False" w971 {
          tunnel: w970 -> [w983 w994]
          tunnel: [w982 w993] -> w969
          tunnel: w966 -> [w981 w992]
          tunnel: [w980 w991] -> w968
          tunnel: w967 -> [w978 w989]
          tunnel: w966 -> [w977 w988]
          frame False {
            n421 = Enqueue Element(queue=w978, element=datalog."Stop Timer", error in (no error)=w977) -> (queue out=w975:refnum<queue>, error out=w974:errorcluster)  [unwired: 1 in, 1 out]
            n422 = Enqueue Element(queue=w983, element=startup_FSM."IDLE", error in (no error)=w981) -> (queue out=w982:refnum<queue>, error out=w980:errorcluster)  [unwired: 1 in, 1 out]
            n423 = Enqueue Element(queue=w975, element=datalog."Read All", error in (no error)=w974) -> ()  [unwired: 1 in, 3 out]
          }
          frame True {
            n424 = Enqueue Element(queue=w989, element=datalog."Read All", error in (no error)=w988) -> (queue out=w986:refnum<queue>, error out=w985:errorcluster)  [unwired: 1 in, 1 out]
            n425 = Enqueue Element(queue=w994, element=startup_FSM."READ", error in (no error)=w992) -> (queue out=w993:refnum<queue>, error out=w991:errorcluster)  [unwired: 1 in, 1 out]
            n426 = Enqueue Element(queue=w986, element=datalog."Start Timer", error in (no error)=w985) -> ()  [unwired: 1 in, 3 out]
          }
        }
      }
    }
    n427 = Wait Until Next ms Multiple(millisecond multiple=u32 10) -> ()  [unwired: 1 out]
    n428 = case shown="No Error" w609 {
      selector: w609 -> [w619 w629]
      tunnel: [w620 w622] -> w611
      tunnel: w607 -> [w620 w630]
      tunnel: [w619 w624] -> w614
      tunnel: w608 -> [w618 w631]
      tunnel: [w618 w623] -> w612
      tunnel: [FALSE TRUE] -> w610
      frame No Error {
      }
      frame Error {
        n429 = Enqueue Element(queue=w631, element=dc_ps_FSM."ERROR", error in (no error)=w629) -> (queue out=w623:refnum<queue>, error out=w626:errorcluster)  [unwired: 1 in, 1 out]
        n430 = Enqueue Element(queue=w630, element=startup_FSM."ERROR", error in (no error)=w629) -> (queue out=w622:refnum<queue>, error out=w625:errorcluster)  [unwired: 1 in, 1 out]
        n431 = Merge Errors(w626, w625) -> (w624:errorcluster)
      }
    }
  }
  n432 = while {
    tunnel: w62 -> [w1008]
    shift-right: [w1004] -> w31
    shift-left: w58 -> [w1009]
    tunnel: w50 -> [w1002]
    tunnel: w40 -> [w1003]
    tunnel: [w997] -> w27
    shift-right: [w995] -> _
    shift-left: dbl[] [] -> [w996]
    stop <- w999 stop-if-true
    # "Serial Communication\nCommands & Events \nConsumer"
    n433 = case shown="No Error" w1009 {
      selector: w1009 -> [w1106 w1112]
      tunnel: w1008 -> [w1107 w1109]
      tunnel: [w1105 w1112] -> w1007
      tunnel: [w1104 w1109] -> w1006
      tunnel: [w1103 startup_FSM."ERROR" ("element")] -> w1005
      tunnel: [w1102 w1111] -> w1001
      tunnel: w1003 -> [w1102 w1111]
      tunnel: [w1101 w1110] -> w1000
      tunnel: w1002 -> [w1101 w1110]
      frame No Error {
        n434 = Dequeue Element(queue=w1107, error in (no error)=w1106) -> (queue out=w1104:refnum<queue>, element=w1103:T8, error out=w1105:errorcluster)  [unwired: 1 in, 1 out]
      }
      frame Error {
      }
    }
    n435 = case shown="\"READ\"" w1005 {
      tunnel: w1007 -> [w1014 w1026 w1029 w1039 w1046 w1069 w1074 w1077 w1082 _ _ _ w1096 w1099]
      tunnel: w1006 -> [_ _ _ _ w1043 _ _ _ _ _ _ _ _ _]
      tunnel: [w1013 _ w1028 w1038 w1045 w1068 w1072 w1076 w1080 _ _ w1093 w1096 w1098] -> w1004
      tunnel: w1001 -> [w1011 _ _ _ w1047 _ _ _ _ _ _ w1095 _ w1100]
      tunnel: w1000 -> [w1016 w1024 w1034 w1040 _ w1071 w1075 w1079 w1083 _ _ w1094 _ _]
      tunnel: [FALSE _ _ _ _ _ _ _ _ _ _ TRUE _ _] -> w999
      tunnel: [w1012 _ _ _ _ _ _ _ _ _ _ _ _ _] -> w997
      tunnel: w996 -> [_ _ _ _ w1042 _ _ _ _ _ _ _ _ _]
      tunnel: [_ _ _ _ w1041 _ _ _ _ _ _ _ _ _] -> w995
      frame "INIT", Default {
        n436 = vi-ref "serial_connection_FSM_2.vi"() -> (w1019:refnum<vi>)
        n437 = Open VI Reference(type specifier VI Refnum (for type only)=w1019, vi path=path "C:/Users/anton/myUnisannio/magistrale/MAPI/esame/labview/serial_connection_FSM_2.vi", options=128) -> (vi reference=w1020:refnum<vi>, error out=w1015:errorcluster)  [unwired: 3 in]
        n438 = Merge Errors(w1015, w1014) -> (w1010:errorcluster)
        n439 = call-by-ref "Start Asynchronous Call"(reference=w1020, "commands_q"=w1016, "sensor_data_q"=w1011, "error in (no error)"=w1010) -> (reference out=w1012:refnum<vi>, error out=w1013:errorcluster)  [unwired: 13 in, 1 out]
      }
      frame "CHANGE BAUD" {
        n440 = Concatenate Strings("SET:BAUD ", "BAUD") -> (w1023:string)
        n441 = Enqueue Element(queue=w1024, element=w1023, error in (no error)=w1026) -> ()  [unwired: 1 in, 3 out]
      }
      frame "CHANGE SAMP. FREQ." {
        n442 = Number To Fractional String(number="SAMP. FREQ. [HZ]", precision (6)=i16 2) -> (F-format string=w1031:string)  [unwired: 2 in]
        n443 = Concatenate Strings("SF " ("string"), w1031) -> (w1030:string)
        n444 = Enqueue Element(queue=w1034, element=w1030, error in (no error)=w1029) -> (error out=w1028:errorcluster)  [unwired: 1 in, 2 out]
      }
      frame "CHANGE PORT" {
        n445 = Concatenate Strings("SET:PORT " ("element"), "SERIAL PORT") -> (w1035:string)
        n446 = Enqueue Element(queue=w1040, element=w1035, error in (no error)=w1039) -> (error out=w1038:errorcluster)  [unwired: 1 in, 2 out]
      }
      frame "READ" {
        n447 = local read "Read Button"() -> (w1044:bool)
        n448 = case shown="True" w1044 {
          tunnel: w1047 -> [_ w1067]
          tunnel: w1046 -> [w1049 w1066]
          tunnel: [w1049 w1065] -> w1045
          tunnel: w1043 -> [_ w1064]
          tunnel: w1042 -> [_ w1053]
          tunnel: [dbl[] [] w1052] -> w1041
          frame False {
          }
          frame True {
            n449 = local read "SAMPLE  COUNT"() -> (w1056:dbl)
            n450 = Enqueue Element(queue=w1064, element=startup_FSM."READ") -> ()  [unwired: 2 in, 3 out]
            n451 = Dequeue Element(queue=w1067, error in (no error)=w1066) -> (element=w1060:string, error out=w1065:errorcluster)  [unwired: 1 in, 2 out]
            n452 = Empty String/Path?(string/path=w1060) -> (empty?=w1059:bool)
            n453 = Select(t=0.0, s=w1059, f=1.0) -> (s? t:f=w1055:dbl)
            n454 = Add(x=w1055, y=w1056) -> (x+y=w1050:dbl)
            n455 = local write "SAMPLE  COUNT"(w1050) -> ()
            n456 = Fract/Exp String To Number(string=w1060) -> (number=w1051:dbl)  [unwired: 3 in, 1 out]
            "flow meas" <- w1051
            n457 = local read "SAMP. FREQ. [HZ]"() -> (w1062:dbl)
            n458 = Build Array (concatenate) "Build Array"(w1053, w1051) -> (w1052:dbl[])
            n459 = Reciprocal(x=w1062) -> (1/x=w1061:dbl)
            n460 = Bundle By Name "Build Waveform"("Y"=w1052, "dt"=w1061) -> (→"Digital Flow Measurements":waveform(dbl))  [unwired: 1 in]
          }
        }
      }
      frame "DISCONNECT" {
        n461 = Enqueue Element(queue=w1071, element="DISCONNECT", error in (no error)=w1069) -> (error out=w1068:errorcluster)  [unwired: 1 in, 2 out]
      }
      frame "CONNECT" {
        n462 = Enqueue Element(queue=w1075, element="CONNECT", error in (no error)=w1074) -> (error out=w1072:errorcluster)  [unwired: 1 in, 2 out]
      }
      frame "OUTPUT OFF" {
        n463 = Enqueue Element(queue=w1079, element="OUTPUT OFF", error in (no error)=w1077) -> (error out=w1076:errorcluster)  [unwired: 1 in, 2 out]
      }
      frame "OUTPUT ON" {
        n464 = Enqueue Element(queue=w1083, element="OUTPUT ON", error in (no error)=w1082) -> (error out=w1080:errorcluster)  [unwired: 1 in, 2 out]
      }
      frame "MEAS_UNIT_L" {
        n465 = local read "Digital Flow Measurements"() -> (w1085:waveform(dbl))
        n466 = Divide(x=w1085, y=1000.0) -> (x/y=w1084:waveform(dbl))
        n467 = local write "Digital Flow Measurements"(w1084) -> ()
      }
      frame "MEAS_UNIT_mL" {
        n468 = local read "Digital Flow Measurements"() -> (w1089:waveform(dbl))
        n469 = Multiply(x=w1089, y=1000.0) -> (x*y=w1087:waveform(dbl))
        n470 = local write "Digital Flow Measurements"(w1087) -> ()
      }
      frame "ERROR" {
        n471 = Release Queue(queue=w1094) -> (error out=w1091:errorcluster)  [unwired: 2 in, 2 out]
        n472 = Release Queue(queue=w1095) -> (error out=w1092:errorcluster)  [unwired: 2 in, 2 out]
        n473 = Merge Errors(w1092, w1091) -> (w1093:errorcluster)
      }
      frame "IDLE" {
      }
      frame "CLEAR BUFF" {
        n474 = Flush Queue(queue=w1100, error in (no error)=w1099) -> (error out=w1098:errorcluster)  [unwired: 2 out]
        n475 = local write "SAMPLE  COUNT"(0.0) -> ()
        n476 = invoke on="Digital Flow Measurements" class="WFGraph (strict)" method="Reinit To Default"() -> ()  [unwired: 3 in, 3 out]
      }
    }
    n477 = Wait Until Next ms Multiple(millisecond multiple=u32 20) -> ()  [unwired: 1 out]
  }
  n478 = while {
    tunnel: w5 -> [w1121]
    tunnel: w7 -> [w1123]
    tunnel: w6 -> [w1122]
    tunnel: w4 -> [w1119]
    tunnel: w3 -> [w1116]
    tunnel: w2 -> [w1117]
    stop <- w1113 stop-if-true
    # "DAQ \nEvents & Commands\nConsumer"
    n479 = Merge Errors(w1123, w1122, w1117) -> (w1124:errorcluster)
    n480 = case shown="No Error" w1124 {
      selector: w1124 -> [w1139 _]
      tunnel: w1121 -> [w1140 _]
      tunnel: [w1138 _] -> w1114
      tunnel: [w1137 _] -> w1120
      tunnel: [w1136 _] -> w1118
      tunnel: w1119 -> [w1136 _]
      tunnel: [w1135 _] -> w1115
      tunnel: w1116 -> [w1135 _]
      frame No Error {
        n481 = Dequeue Element(queue=w1140, error in (no error)=w1139) -> (element=w1137:T3, error out=w1138:errorcluster)  [unwired: 1 in, 2 out]
      }
      frame Error {
      }
    }
    n482 = case shown="\"Initialize\"" w1120 {
      tunnel: w1118 -> [_ w1130]
      tunnel: w1115 -> [_ w1131]
      tunnel: w1114 -> [_ w1127]
      tunnel: [_ FALSE] -> w1113
      frame "", Default {
      }
      frame "Initialize" {
        n483 = vi-ref "daq_FSM.vi"() -> (w1134:refnum<vi>)
        n484 = Open VI Reference(vi path=path "C:/Users/anton/myUnisannio/magistrale/MAPI/esame/labview/daq_FSM.vi", options=128) -> (error out=w1128:errorcluster)  [unwired: 4 in, 1 out]
        n485 = Merge Errors(w1128, w1127) -> (w1129:errorcluster)
        n486 = call-by-ref "Start Asynchronous Call"(reference=w1134, error in=w1128, 8:"error in (no error)"=w1129, "Measures"=w1131, "Commands"=w1130) -> ()  [unwired: 9 in, 2 out]
      }
    }
    n487 = Wait Until Next ms Multiple(millisecond multiple=u32 20) -> ()  [unwired: 1 out]
  }
  n488 = Close Reference(reference=w27) -> ()  [unwired: 1 in, 1 out]
  n489 = Release Queue(queue=w36, error in (no error)=w34) -> (error out=w33:errorcluster)  [unwired: 1 in, 2 out]
  n490 = Release Queue(queue=w35, error in (no error)=w34) -> (error out=w32:errorcluster)  [unwired: 1 in, 2 out]
  n491 = Merge Errors(w33, w32, w31, w30, w13, w12) -> (w29:errorcluster)
  n492 = call <vilib>:"Simple Error Handler.vi"("error in (no error)"=w29) -> ()  [unwired: 4 in, 5 out]
